vi "_old_Load_SetList_Convert_v4.0_to_v4.1.vi"(0 "Path":path) -> (1 "Procedure Name":string="IBS_PICameraTest_29Sep04", 2 "Paramaters":T1={"Master PB Staging List"=[{"Output Bits"=[], "Delay (s)"="", "String"="", "Halt?"=FALSE}, {"Output Bits"=[], "Delay (s)"="", "String"="", "Halt?"=FALSE}, {"Output Bits"=[], "Delay (s)"="", "String"="", "Halt?"=FALSE}, {"Output Bits"=[], "Delay (s)"="", "String"="", "Halt?"=FALSE}, {"Output Bits"=[], "Delay (s)"="", "String"="", "Halt?"=FALSE}, {"Output Bits"=[], "Delay (s)"="", "String"="", "Halt?"=FALSE}, {"Output Bits"=[], "Delay (s)"="", "String"="", "Halt?"=FALSE}, {"Output Bits"=[], "Delay (s)"="", "String"="", "Halt?"=FALSE}, {"Output Bits"=[], "Delay (s)"="", "String"="", "Halt?"=FALSE}, {"Output Bits"=[], "Delay (s)"="", "String"="", "Halt?"=FALSE}, {"Output Bits"=[], "Delay (s)"="", "String"="", "Halt?"=FALSE}, {"Output Bits"=[], "Delay (s)"="", "String"="", "Halt?"=FALSE}, {"Output Bits"=[], "Delay (s)"="", "String"="", "Halt?"=FALSE}, {"Output Bits"=[], "Delay (s)"="", "String"="", "Halt?"=FALSE}, {"Output Bits"=[], "Delay (s)"="", "String"="", "Halt?"=FALSE}, {"Output Bits"=[], "Delay (s)"="", "String"="", "Halt?"=FALSE}, {"Output Bits"=[], "Delay (s)"="", "String"="", "Halt?"=FALSE}, {"Output Bits"=[], "Delay (s)"="", "String"="", "Halt?"=FALSE}, {"Output Bits"=[], "Delay (s)"="", "String"="", "Halt?"=FALSE}, {"Output Bits"=[], "Delay (s)"="", "String"="", "Halt?"=FALSE}, {"Output Bits"=[], "Delay (s)"="", "String"="", "Halt?"=FALSE}, {"Output Bits"=[], "Delay (s)"="", "String"="", "Halt?"=FALSE}, {"Output Bits"=[], "Delay (s)"="", "String"="", "Halt?"=FALSE}, {"Output Bits"=[], "Delay (s)"="", "String"="", "Halt?"=FALSE}, {"Output Bits"=[], "Delay (s)"="", "String"="", "Halt?"=FALSE}, {"Output Bits"=[], "Delay (s)"="", "String"="", "Halt?"=FALSE}, {"Output Bits"=[], "Delay (s)"="", "String"="", "Halt?"=FALSE}, {"Output Bits"=[], "Delay (s)"="", "String"="", "Halt?"=FALSE}, {"Output Bits"=[], "Delay (s)"="", "String"="", "Halt?"=FALSE}, {"Output Bits"=[], "Delay (s)"="", "String"="", "Halt?"=FALSE}, {"Output Bits"=[], "Delay (s)"="", "String"="", "Halt?"=FALSE}, {"Output Bits"=[], "Delay (s)"="", "String"="", "Halt?"=FALSE}, {"Output Bits"=[], "Delay (s)"="", "String"="", "Halt?"=FALSE}, {"Output Bits"=[], "Delay (s)"="", "String"="", "Halt?"=FALSE}, {"Output Bits"=[], "Delay (s)"="", "String"="", "Halt?"=FALSE}, {"Output Bits"=[], "Delay (s)"="", "String"="", "Halt?"=FALSE}, {"Output Bits"=[], "Delay (s)"="", "String"="", "Halt?"=FALSE}, {"Output Bits"=[], "Delay (s)"="", "String"="", "Halt?"=FALSE}, {"Output Bits"=[], "Delay (s)"="", "String"="", "Halt?"=FALSE}, {"Output Bits"=[], "Delay (s)"="", "String"="", "Halt?"=FALSE}, {"Output Bits"=[], "Delay (s)"="", "String"="", "Halt?"=FALSE}, {"Output Bits"=[], "Delay (s)"="", "String"="", "Halt?"=FALSE}, {"Output Bits"=[], "Delay (s)"="", "String"="", "Halt?"=FALSE}, {"Output Bits"=[], "Delay (s)"="", "String"="", "Halt?"=FALSE}], "Slave PB Staging List"=[{"Output Bits"=[], "Delay (s)"="", "String"="", "Halt?"=FALSE}, {"Output Bits"=[], "Delay (s)"="", "String"="", "Halt?"=FALSE}, {"Output Bits"=[], "Delay (s)"="", "String"="", "Halt?"=FALSE}, {"Output Bits"=[], "Delay (s)"="", "String"="", "Halt?"=FALSE}, {"Output Bits"=[], "Delay (s)"="", "String"="", "Halt?"=FALSE}, {"Output Bits"=[], "Delay (s)"="", "String"="", "Halt?"=FALSE}, {"Output Bits"=[], "Delay (s)"="", "String"="", "Halt?"=FALSE}, {"Output Bits"=[], "Delay (s)"="", "String"="", "Halt?"=FALSE}, {"Output Bits"=[], "Delay (s)"="", "String"="", "Halt?"=FALSE}, {"Output Bits"=[], "Delay (s)"="", "String"="", "Halt?"=FALSE}, {"Output Bits"=[], "Delay (s)"="", "String"="", "Halt?"=FALSE}, {"Output Bits"=[], "Delay (s)"="", "String"="", "Halt?"=FALSE}, {"Output Bits"=[], "Delay (s)"="", "String"="", "Halt?"=FALSE}, {"Output Bits"=[], "Delay (s)"="", "String"="", "Halt?"=FALSE}, {"Output Bits"=[], "Delay (s)"="", "String"="", "Halt?"=FALSE}, {"Output Bits"=[], "Delay (s)"="", "String"="", "Halt?"=FALSE}, {"Output Bits"=[], "Delay (s)"="", "String"="", "Halt?"=FALSE}, {"Output Bits"=[], "Delay (s)"="", "String"="", "Halt?"=FALSE}, {"Output Bits"=[], "Delay (s)"="", "String"="", "Halt?"=FALSE}, {"Output Bits"=[], "Delay (s)"="", "String"="", "Halt?"=FALSE}, {"Output Bits"=[], "Delay (s)"="", "String"="", "Halt?"=FALSE}, {"Output Bits"=[], "Delay (s)"="", "String"="", "Halt?"=FALSE}, {"Output Bits"=[], "Delay (s)"="", "String"="", "Halt?"=FALSE}, {"Output Bits"=[], "Delay (s)"="", "String"="", "Halt?"=FALSE}, {"Output Bits"=[], "Delay (s)"="", "String"="", "Halt?"=FALSE}, {"Output Bits"=[], "Delay (s)"="", "String"="", "Halt?"=FALSE}, {"Output Bits"=[], "Delay (s)"="", "String"="", "Halt?"=FALSE}, {"Output Bits"=[], "Delay (s)"="", "String"="", "Halt?"=FALSE}, {"Output Bits"=[], "Delay (s)"="", "String"="", "Halt?"=FALSE}, {"Output Bits"=[], "Delay (s)"="", "String"="", "Halt?"=FALSE}, {"Output Bits"=[], "Delay (s)"="", "String"="", "Halt?"=FALSE}, {"Output Bits"=[], "Delay (s)"="", "String"="", "Halt?"=FALSE}, {"Output Bits"=[], "Delay (s)"="", "String"="", "Halt?"=FALSE}, {"Output Bits"=[], "Delay (s)"="", "String"="", "Halt?"=FALSE}, {"Output Bits"=[], "Delay (s)"="", "String"="", "Halt?"=FALSE}, {"Output Bits"=[], "Delay (s)"="", "String"="", "Halt?"=FALSE}, {"Output Bits"=[], "Delay (s)"="", "String"="", "Halt?"=FALSE}, {"Output Bits"=[], "Delay (s)"="", "String"="", "Halt?"=FALSE}, {"Output Bits"=[], "Delay (s)"="", "String"="", "Halt?"=FALSE}, {"Output Bits"=[], "Delay (s)"="", "String"="", "Halt?"=FALSE}, {"Output Bits"=[], "Delay (s)"="", "String"="", "Halt?"=FALSE}, {"Output Bits"=[], "Delay (s)"="", "String"="", "Halt?"=FALSE}, {"Output Bits"=[], "Delay (s)"="", "String"="", "Halt?"=FALSE}, {"Output Bits"=[], "Delay (s)"="", "String"="", "Halt?"=FALSE}], "Novatech Ramps"=[{"Ramp Channels"=[], "2 Freq. [MHz]"="", "2 Power [dBm]"="", "3 Freq. [MHz]"="", "3 Power [dBm]"="", "Serial Port"=""}, {"Ramp Channels"=[], "2 Freq. [MHz]"="", "2 Power [dBm]"="", "3 Freq. [MHz]"="", "3 Power [dBm]"="", "Serial Port"=""}, {"Ramp Channels"=[], "2 Freq. [MHz]"="", "2 Power [dBm]"="", "3 Freq. [MHz]"="", "3 Power [dBm]"="", "Serial Port"=""}, {"Ramp Channels"=[], "2 Freq. [MHz]"="", "2 Power [dBm]"="", "3 Freq. [MHz]"="", "3 Power [dBm]"="", "Serial Port"=""}, {"Ramp Channels"=[], "2 Freq. [MHz]"="", "2 Power [dBm]"="", "3 Freq. [MHz]"="", "3 Power [dBm]"="", "Serial Port"=""}, {"Ramp Channels"=[], "2 Freq. [MHz]"="", "2 Power [dBm]"="", "3 Freq. [MHz]"="", "3 Power [dBm]"="", "Serial Port"=""}, {"Ramp Channels"=[], "2 Freq. [MHz]"="", "2 Power [dBm]"="", "3 Freq. [MHz]"="", "3 Power [dBm]"="", "Serial Port"=""}], "Sequencing Info"=[{"Start"=0.0, "End"=2.11, "Sequenced Data"=[], "Inform\nIgor?"=FALSE, "Computed Step Size"=0.0, "Procedure Variable"="", "Default"=2.11, "Steps"=0}], "SRS Ramps"=[{"lattice ramp"=[{"dt"="", "formula"=""}, {"dt"="", "formula"=""}, {"dt"="", "formula"=""}], "Output"=[{"Time Values"=[0.0, 0.002, 0.004, 0.006, 0.008, 0.01, 0.012, 0.014, 0.016, 0.018000000000000002, 0.02, 0.022, 0.024, 0.026000000000000002, 0.028, 0.03, 0.032, 0.034, 0.036000000000000004, 0.038, 0.04, 0.042, 0.044, 0.046, 0.048, 0.05, 0.052000000000000005, 0.054, 0.056, 0.058, 0.06, 0.062, 0.064, 0.066, 0.068, 0.07, 0.07200000000000001, 0.074, 0.076, 0.078, 0.08, 0.082, 0.084, 0.08600000000000001, 0.088, 0.09, 0.092, 0.094, 0.096, 0.098, 0.1, 0.10200000000000001, 0.10400000000000001, 0.106, 0.108, 0.11, 0.112, 0.114, 0.116, 0.11800000000000001, 0.12, 0.122, 0.124, 0.126, 0.128, 0.13, 0.132, 0.134, 0.136, 0.138, 0.14, 0.14200000000000002, 0.14400000000000002, 0.146, 0.148, 0.15, 0.152, 0.154, 0.156, 0.158, 0.16, 0.162, 0.164, 0.166, 0.168, 0.17, 0.17200000000000001, 0.17400000000000002, 0.176, 0.178, 0.18, 0.182, 0.184, 0.186, 0.188, 0.19, 0.192, 0.194, 0.196, 0.198, 0.2, 0.6000000000000001, 0.6000000000000001, 0.6002000000000001, 0.6004, 0.6006000000000001, 0.6008000000000001, 0.6010000000000001, 0.6012000000000001, 0.6014, 0.6016000000000001, 0.6018000000000001, 0.6020000000000001, 0.6022000000000001, 0.6024, 0.6026000000000001, 0.6028000000000001, 0.6030000000000001, 0.6032000000000001, 0.6034, 0.6036000000000001, 0.6038000000000001, 0.6040000000000001, 0.6042000000000001, 0.6044, 0.6046000000000001, 0.6048000000000001, 0.6050000000000001, 0.6052000000000001, 0.6054, 0.6056000000000001, 0.6058000000000001, 0.6060000000000001, 0.6062000000000001, 0.6064, 0.6066000000000001, 0.6068000000000001, 0.6070000000000001, 0.6072000000000001, 0.6074, 0.6076000000000001, 0.6078000000000001, 0.6080000000000001, 0.6082000000000001, 0.6084, 0.6086000000000001, 0.6088000000000001, 0.6090000000000001, 0.6092000000000001, 0.6094, 0.6096000000000001, 0.6098000000000001, 0.6100000000000001, 0.6102000000000001, 0.6104, 0.6106000000000001, 0.6108000000000001, 0.6110000000000001, 0.6112000000000001, 0.6114, 0.6116000000000001, 0.6118000000000001, 0.6120000000000001, 0.6122000000000001, 0.6124, 0.6126, 0.6128000000000001, 0.6130000000000001, 0.6132000000000001, 0.6134000000000001, 0.6136000000000001, 0.6138000000000001, 0.6140000000000001, 0.6142000000000001, 0.6144000000000001, 0.6146, 0.6148000000000001, 0.6150000000000001, 0.6152000000000001, 0.6154000000000001, 0.6156, 0.6158000000000001, 0.6160000000000001, 0.6162000000000001, 0.6164000000000001, 0.6166, 0.6168000000000001, 0.6170000000000001, 0.6172000000000001, 0.6174000000000001, 0.6176, 0.6178000000000001, 0.6180000000000001, 0.6182000000000001, 0.6184000000000001, 0.6186, 0.6188000000000001, 0.6190000000000001, 0.6192000000000001, 0.6194000000000001, 0.6196, 0.6198000000000001, 0.6200000000000001, 0.6202000000000001, 0.6212000000000001], array[205 elements]}, {"Time Values"=[0.0, 0.002, 0.004, 0.006, 0.008, 0.01, 0.012, 0.014, 0.016, 0.018000000000000002, 0.02, 0.022, 0.024, 0.026000000000000002, 0.028, 0.03, 0.032, 0.034, 0.036000000000000004, 0.038, 0.04, 0.042, 0.044, 0.046, 0.048, 0.05, 0.052000000000000005, 0.054, 0.056, 0.058, 0.06, 0.062, 0.064, 0.066, 0.068, 0.07, 0.07200000000000001, 0.074, 0.076, 0.078, 0.08, 0.082, 0.084, 0.08600000000000001, 0.088, 0.09, 0.092, 0.094, 0.096, 0.098, 0.1, 0.10200000000000001, 0.10400000000000001, 0.106, 0.108, 0.11, 0.112, 0.114, 0.116, 0.11800000000000001, 0.12, 0.122, 0.124, 0.126, 0.128, 0.13, 0.132, 0.134, 0.136, 0.138, 0.14, 0.14200000000000002, 0.14400000000000002, 0.146, 0.148, 0.15, 0.152, 0.154, 0.156, 0.158, 0.16, 0.162, 0.164, 0.166, 0.168, 0.17, 0.17200000000000001, 0.17400000000000002, 0.176, 0.178, 0.18, 0.182, 0.184, 0.186, 0.188, 0.19, 0.192, 0.194, 0.196, 0.198, 0.2, 0.6000000000000001, 0.6000000000000001, 0.6002000000000001, 0.6004, 0.6006000000000001, 0.6008000000000001, 0.6010000000000001, 0.6012000000000001, 0.6014, 0.6016000000000001, 0.6018000000000001, 0.6020000000000001, 0.6022000000000001, 0.6024, 0.6026000000000001, 0.6028000000000001, 0.6030000000000001, 0.6032000000000001, 0.6034, 0.6036000000000001, 0.6038000000000001, 0.6040000000000001, 0.6042000000000001, 0.6044, 0.6046000000000001, 0.6048000000000001, 0.6050000000000001, 0.6052000000000001, 0.6054, 0.6056000000000001, 0.6058000000000001, 0.6060000000000001, 0.6062000000000001, 0.6064, 0.6066000000000001, 0.6068000000000001, 0.6070000000000001, 0.6072000000000001, 0.6074, 0.6076000000000001, 0.6078000000000001, 0.6080000000000001, 0.6082000000000001, 0.6084, 0.6086000000000001, 0.6088000000000001, 0.6090000000000001, 0.6092000000000001, 0.6094, 0.6096000000000001, 0.6098000000000001, 0.6100000000000001, 0.6102000000000001, 0.6104, 0.6106000000000001, 0.6108000000000001, 0.6110000000000001, 0.6112000000000001, 0.6114, 0.6116000000000001, 0.6118000000000001, 0.6120000000000001, 0.6122000000000001, 0.6124, 0.6126, 0.6128000000000001, 0.6130000000000001, 0.6132000000000001, 0.6134000000000001, 0.6136000000000001, 0.6138000000000001, 0.6140000000000001, 0.6142000000000001, 0.6144000000000001, 0.6146, 0.6148000000000001, 0.6150000000000001, 0.6152000000000001, 0.6154000000000001, 0.6156, 0.6158000000000001, 0.6160000000000001, 0.6162000000000001, 0.6164000000000001, 0.6166, 0.6168000000000001, 0.6170000000000001, 0.6172000000000001, 0.6174000000000001, 0.6176, 0.6178000000000001, 0.6180000000000001, 0.6182000000000001, 0.6184000000000001, 0.6186, 0.6188000000000001, 0.6190000000000001, 0.6192000000000001, 0.6194000000000001, 0.6196, 0.6198000000000001, 0.6200000000000001, 0.6202000000000001, 0.6212000000000001], array[205 elements]}], "SRS Selection"=enum."1550 Vertical"}, {"lattice ramp"=[{"dt"="", "formula"=""}], "Output"=[{"Time Values"=[0.0, 0.002, 0.004, 0.006, 0.008, 0.01, 0.012, 0.014, 0.016, 0.018000000000000002, 0.02, 0.022, 0.024, 0.026000000000000002, 0.028, 0.03, 0.032, 0.034, 0.036000000000000004, 0.038, 0.04, 0.042, 0.044, 0.046, 0.048, 0.05, 0.052000000000000005, 0.054, 0.056, 0.058, 0.06, 0.062, 0.064, 0.066, 0.068, 0.07, 0.07200000000000001, 0.074, 0.076, 0.078, 0.08, 0.082, 0.084, 0.08600000000000001, 0.088, 0.09, 0.092, 0.094, 0.096, 0.098, 0.1, 0.10200000000000001, 0.10400000000000001, 0.106, 0.108, 0.11, 0.112, 0.114, 0.116, 0.11800000000000001, 0.12, 0.122, 0.124, 0.126, 0.128, 0.13, 0.132, 0.134, 0.136, 0.138, 0.14, 0.14200000000000002, 0.14400000000000002, 0.146, 0.148, 0.15, 0.152, 0.154, 0.156, 0.158, 0.16, 0.162, 0.164, 0.166, 0.168, 0.17, 0.17200000000000001, 0.17400000000000002, 0.176, 0.178, 0.18, 0.182, 0.184, 0.186, 0.188, 0.19, 0.192, 0.194, 0.196, 0.198, 0.2, 0.6000000000000001, 0.6000000000000001, 0.6002000000000001, 0.6004, 0.6006000000000001, 0.6008000000000001, 0.6010000000000001, 0.6012000000000001, 0.6014, 0.6016000000000001, 0.6018000000000001, 0.6020000000000001, 0.6022000000000001, 0.6024, 0.6026000000000001, 0.6028000000000001, 0.6030000000000001, 0.6032000000000001, 0.6034, 0.6036000000000001, 0.6038000000000001, 0.6040000000000001, 0.6042000000000001, 0.6044, 0.6046000000000001, 0.6048000000000001, 0.6050000000000001, 0.6052000000000001, 0.6054, 0.6056000000000001, 0.6058000000000001, 0.6060000000000001, 0.6062000000000001, 0.6064, 0.6066000000000001, 0.6068000000000001, 0.6070000000000001, 0.6072000000000001, 0.6074, 0.6076000000000001, 0.6078000000000001, 0.6080000000000001, 0.6082000000000001, 0.6084, 0.6086000000000001, 0.6088000000000001, 0.6090000000000001, 0.6092000000000001, 0.6094, 0.6096000000000001, 0.6098000000000001, 0.6100000000000001, 0.6102000000000001, 0.6104, 0.6106000000000001, 0.6108000000000001, 0.6110000000000001, 0.6112000000000001, 0.6114, 0.6116000000000001, 0.6118000000000001, 0.6120000000000001, 0.6122000000000001, 0.6124, 0.6126, 0.6128000000000001, 0.6130000000000001, 0.6132000000000001, 0.6134000000000001, 0.6136000000000001, 0.6138000000000001, 0.6140000000000001, 0.6142000000000001, 0.6144000000000001, 0.6146, 0.6148000000000001, 0.6150000000000001, 0.6152000000000001, 0.6154000000000001, 0.6156, 0.6158000000000001, 0.6160000000000001, 0.6162000000000001, 0.6164000000000001, 0.6166, 0.6168000000000001, 0.6170000000000001, 0.6172000000000001, 0.6174000000000001, 0.6176, 0.6178000000000001, 0.6180000000000001, 0.6182000000000001, 0.6184000000000001, 0.6186, 0.6188000000000001, 0.6190000000000001, 0.6192000000000001, 0.6194000000000001, 0.6196, 0.6198000000000001, 0.6200000000000001, 0.6202000000000001, 0.6212000000000001], array[205 elements]}, {"Time Values"=[0.0, 0.002, 0.004, 0.006, 0.008, 0.01, 0.012, 0.014, 0.016, 0.018000000000000002, 0.02, 0.022, 0.024, 0.026000000000000002, 0.028, 0.03, 0.032, 0.034, 0.036000000000000004, 0.038, 0.04, 0.042, 0.044, 0.046, 0.048, 0.05, 0.052000000000000005, 0.054, 0.056, 0.058, 0.06, 0.062, 0.064, 0.066, 0.068, 0.07, 0.07200000000000001, 0.074, 0.076, 0.078, 0.08, 0.082, 0.084, 0.08600000000000001, 0.088, 0.09, 0.092, 0.094, 0.096, 0.098, 0.1, 0.10200000000000001, 0.10400000000000001, 0.106, 0.108, 0.11, 0.112, 0.114, 0.116, 0.11800000000000001, 0.12, 0.122, 0.124, 0.126, 0.128, 0.13, 0.132, 0.134, 0.136, 0.138, 0.14, 0.14200000000000002, 0.14400000000000002, 0.146, 0.148, 0.15, 0.152, 0.154, 0.156, 0.158, 0.16, 0.162, 0.164, 0.166, 0.168, 0.17, 0.17200000000000001, 0.17400000000000002, 0.176, 0.178, 0.18, 0.182, 0.184, 0.186, 0.188, 0.19, 0.192, 0.194, 0.196, 0.198, 0.2, 0.6000000000000001, 0.6000000000000001, 0.6002000000000001, 0.6004, 0.6006000000000001, 0.6008000000000001, 0.6010000000000001, 0.6012000000000001, 0.6014, 0.6016000000000001, 0.6018000000000001, 0.6020000000000001, 0.6022000000000001, 0.6024, 0.6026000000000001, 0.6028000000000001, 0.6030000000000001, 0.6032000000000001, 0.6034, 0.6036000000000001, 0.6038000000000001, 0.6040000000000001, 0.6042000000000001, 0.6044, 0.6046000000000001, 0.6048000000000001, 0.6050000000000001, 0.6052000000000001, 0.6054, 0.6056000000000001, 0.6058000000000001, 0.6060000000000001, 0.6062000000000001, 0.6064, 0.6066000000000001, 0.6068000000000001, 0.6070000000000001, 0.6072000000000001, 0.6074, 0.6076000000000001, 0.6078000000000001, 0.6080000000000001, 0.6082000000000001, 0.6084, 0.6086000000000001, 0.6088000000000001, 0.6090000000000001, 0.6092000000000001, 0.6094, 0.6096000000000001, 0.6098000000000001, 0.6100000000000001, 0.6102000000000001, 0.6104, 0.6106000000000001, 0.6108000000000001, 0.6110000000000001, 0.6112000000000001, 0.6114, 0.6116000000000001, 0.6118000000000001, 0.6120000000000001, 0.6122000000000001, 0.6124, 0.6126, 0.6128000000000001, 0.6130000000000001, 0.6132000000000001, 0.6134000000000001, 0.6136000000000001, 0.6138000000000001, 0.6140000000000001, 0.6142000000000001, 0.6144000000000001, 0.6146, 0.6148000000000001, 0.6150000000000001, 0.6152000000000001, 0.6154000000000001, 0.6156, 0.6158000000000001, 0.6160000000000001, 0.6162000000000001, 0.6164000000000001, 0.6166, 0.6168000000000001, 0.6170000000000001, 0.6172000000000001, 0.6174000000000001, 0.6176, 0.6178000000000001, 0.6180000000000001, 0.6182000000000001, 0.6184000000000001, 0.6186, 0.6188000000000001, 0.6190000000000001, 0.6192000000000001, 0.6194000000000001, 0.6196, 0.6198000000000001, 0.6200000000000001, 0.6202000000000001, 0.6212000000000001], array[205 elements]}], "SRS Selection"=enum."1550 Vertical"}], "Master AO Ramp List"=[{"Ramp index"=10, "Ramp time [s]"="", "Step size [s]"=1000.0, "Ramp Array"=[], "Output Bits"=[]}, {"Ramp index"=10, "Ramp time [s]"="", "Step size [s]"=1000.0, "Ramp Array"=[], "Output Bits"=[]}], "Slave AO Ramp List"=[{"Ramp index"=10, "Ramp time [s]"="", "Step size [s]"=1000.0, "Ramp Array"=[], "Output Bits"=[]}, {"Ramp index"=10, "Ramp time [s]"="", "Step size [s]"=1000.0, "Ramp Array"=[], "Output Bits"=[]}], "Master Novatech Ramp List"=[], "Static Variables"=[], "DDS Ramp List"=[]} {"Sequencing Info"."Steps" min=2; "Sequencing Info"."Default" format="%#.7p"; "Sequencing Info"."Computed Step Size" format="%#.7p"; "Sequencing Info"."Sequenced Data" format="%.2e"; "Sequencing Info"."End" format="%#.7p"; "Sequencing Info"."Start" format="%#.7p"})   [LabVIEW 2013]
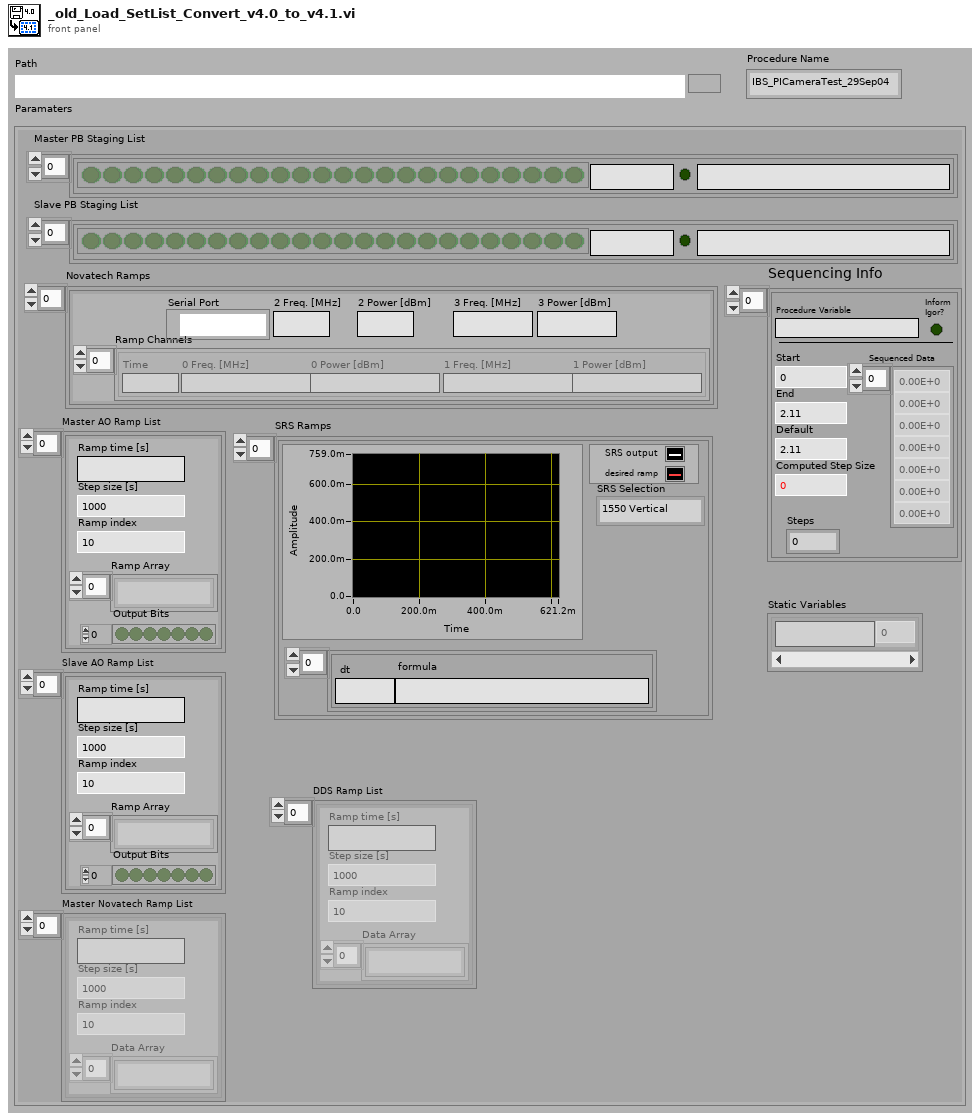
[diagram p1: front panel]
types:
  T1 = cluster{"Master PB Staging List":cluster{"Output Bits":bool[], "Delay (s)":string, "String":string, "Halt?":bool}[], "Slave PB Staging List":cluster{"Output Bits":bool[], "Delay (s)":string, "String":string, "Halt?":bool}[], "Novatech Ramps":cluster{"Ramp Channels":cluster{"Time":string, "0 Freq. [MHz]":string, "0 Power [dBm]":string, "1 Freq. [MHz]":string, "1 Power [dBm]":string}[], "2 Freq. [MHz]":string, "2 Power [dBm]":string, "3 Freq. [MHz]":string, "3 Power [dBm]":string, "Serial Port":refnum<visa-resource-name>}[], "Sequencing Info":cluster{"Start":dbl, "End":dbl, "Sequenced Data":dbl[], "Inform\nIgor?":bool, "Computed Step Size":dbl, "Procedure Variable":string, "Default":dbl, "Steps":i32}[], "SRS Ramps":cluster{"lattice ramp":cluster{"dt":string, "formula":string}[], "Output":cluster{"Time Values":dbl[], dbl[]}[], "SRS Selection":enum16{"1550 Vertical", "Bragg Agilent", "Bragg PTS", "Acc. Intensity"}}[], "Master AO Ramp List":cluster{"Ramp index":u32, "Ramp time [s]":string, "Step size [s]":dbl, "Ramp Array":string[], "Output Bits":bool[]}[], "Slave AO Ramp List":cluster{"Ramp index":u32, "Ramp time [s]":string, "Step size [s]":dbl, "Ramp Array":string[], "Output Bits":bool[]}[], "Master Novatech Ramp List":cluster{"Ramp index":u32, "Ramp time [s]":string, "Step size [s]":dbl, "Data Array":string[]}[], "Static Variables":cluster{"Procedure variable":string, "Value":dbl}[], "DDS Ramp List":cluster{"Ramp index":u32, "Ramp time [s]":string, "Step size [s]":dbl, "Data Array":string[]}[]}
  T2 = cluster{"Master PB Staging List":cluster{"Output Bits":bool[], "Delay (s)":string, "String":string, "Halt?":bool}[], "Slave PB Staging List":cluster{"Output Bits":bool[], "Delay (s)":string, "String":string, "Halt?":bool}[], "Novatech Ramps":cluster{"Ramp Channels":cluster{"Time":string, "0 Freq. [MHz]":string, "0 Power [dBm]":string, "1 Freq. [MHz]":string, "1 Power [dBm]":string}[], "2 Freq. [MHz]":string, "2 Power [dBm]":string, "3 Freq. [MHz]":string, "3 Power [dBm]":string, "Serial Port":refnum<visa-resource-name>}[], "Sequencing Info":cluster{"Start":dbl, "End":dbl, "Sequenced Data":dbl[], "Sequence Data Source":bool, "Inform\nIgor?":bool, "Computed Step Size":dbl, "Procedure Variable":string, "Default":dbl}[], "SRS Ramps":cluster{"lattice ramp":cluster{"dt":string, "formula":string}[], "Output":cluster{"Time Values":dbl[], dbl[]}[], "SRS Selection":enum16{"1550 Vertical", "Bragg Agilent", "Bragg PTS", "Acc. Intensity"}}[], "Master AO Ramp List":cluster{"Ramp index":u32, "Ramp time [s]":string, "Step size [s]":dbl, "Ramp Array":string[], "Output Bits":bool[]}[], "Slave AO Ramp List":cluster{"Ramp index":u32, "Ramp time [s]":string, "Step size [s]":dbl, "Ramp Array":string[], "Output Bits":bool[]}[], "Master Novatech Ramp List":cluster{"Ramp index":u32, "Ramp time [s]":string, "Step size [s]":dbl, "Data Array":string[]}[], "Static Variables":cluster{"Procedure variable":string, "Value":dbl}[]}
  T3 = cluster{"Output Bits":bool[], "Delay (s)":string, "String":string, "Halt?":bool}[]
  T4 = cluster{"Ramp index":u32, "Ramp time [s]":string, "Step size [s]":dbl, "Ramp Array":string[], "Output Bits":bool[]}[]
  T5 = cluster{"Ramp index":u32, "Ramp time [s]":string, "Step size [s]":dbl, "Data Array":string[]}[]
  T6 = cluster{"Ramp Channels":cluster{"Time":string, "0 Freq. [MHz]":string, "0 Power [dBm]":string, "1 Freq. [MHz]":string, "1 Power [dBm]":string}[], "2 Freq. [MHz]":string, "2 Power [dBm]":string, "3 Freq. [MHz]":string, "3 Power [dBm]":string, "Serial Port":refnum<visa-resource-name>}[]
  T7 = cluster{"Start":dbl, "End":dbl, "Sequenced Data":dbl[], "Sequence Data Source":bool, "Inform\nIgor?":bool, "Computed Step Size":dbl, "Procedure Variable":string, "Default":dbl}[]
  T8 = cluster{"lattice ramp":cluster{"dt":string, "formula":string}[], "Output":cluster{"Time Values":dbl[], dbl[]}[], "SRS Selection":enum16{"1550 Vertical", "Bragg Agilent", "Bragg PTS", "Acc. Intensity"}}[]
  T9 = cluster{"Procedure variable":string, "Value":dbl}[]
  T10 = cluster{"Ramp index":u32, "Ramp time [s]":string, "Step size [s]":dbl, "Ramp Array":string[], "Output Bits":bool[]}
  T11 = cluster{"Ramp index":u32, "Ramp time [s]":string, "Step size [s]":dbl, "Data Array":string[]}
  T12 = cluster{"Output Bits":bool[], "Delay (s)":string, "String":string, "Halt?":bool}
  T13 = cluster{"Ramp Channels":cluster{"Time":string, "0 Freq. [MHz]":string, "0 Power [dBm]":string, "1 Freq. [MHz]":string, "1 Power [dBm]":string}[], "2 Freq. [MHz]":string, "2 Power [dBm]":string, "3 Freq. [MHz]":string, "3 Power [dBm]":string, "Serial Port":refnum<visa-resource-name>}
  T14 = cluster{"Start":dbl, "End":dbl, "Sequenced Data":dbl[], "Sequence Data Source":bool, "Inform\nIgor?":bool, "Computed Step Size":dbl, "Procedure Variable":string, "Default":dbl}
  T15 = cluster{"Start":dbl, "End":dbl, "Sequenced Data":dbl[], "Inform\nIgor?":bool, "Computed Step Size":dbl, "Procedure Variable":string, "Default":dbl, "Steps":i32}
  T16 = cluster{"Procedure variable":string, "Value":dbl}
  T17 = cluster{"lattice ramp":cluster{"dt":string, "formula":string}[], "Output":cluster{"Time Values":dbl[], dbl[]}[], "SRS Selection":enum16{"1550 Vertical", "Bragg Agilent", "Bragg PTS", "Acc. Intensity"}}
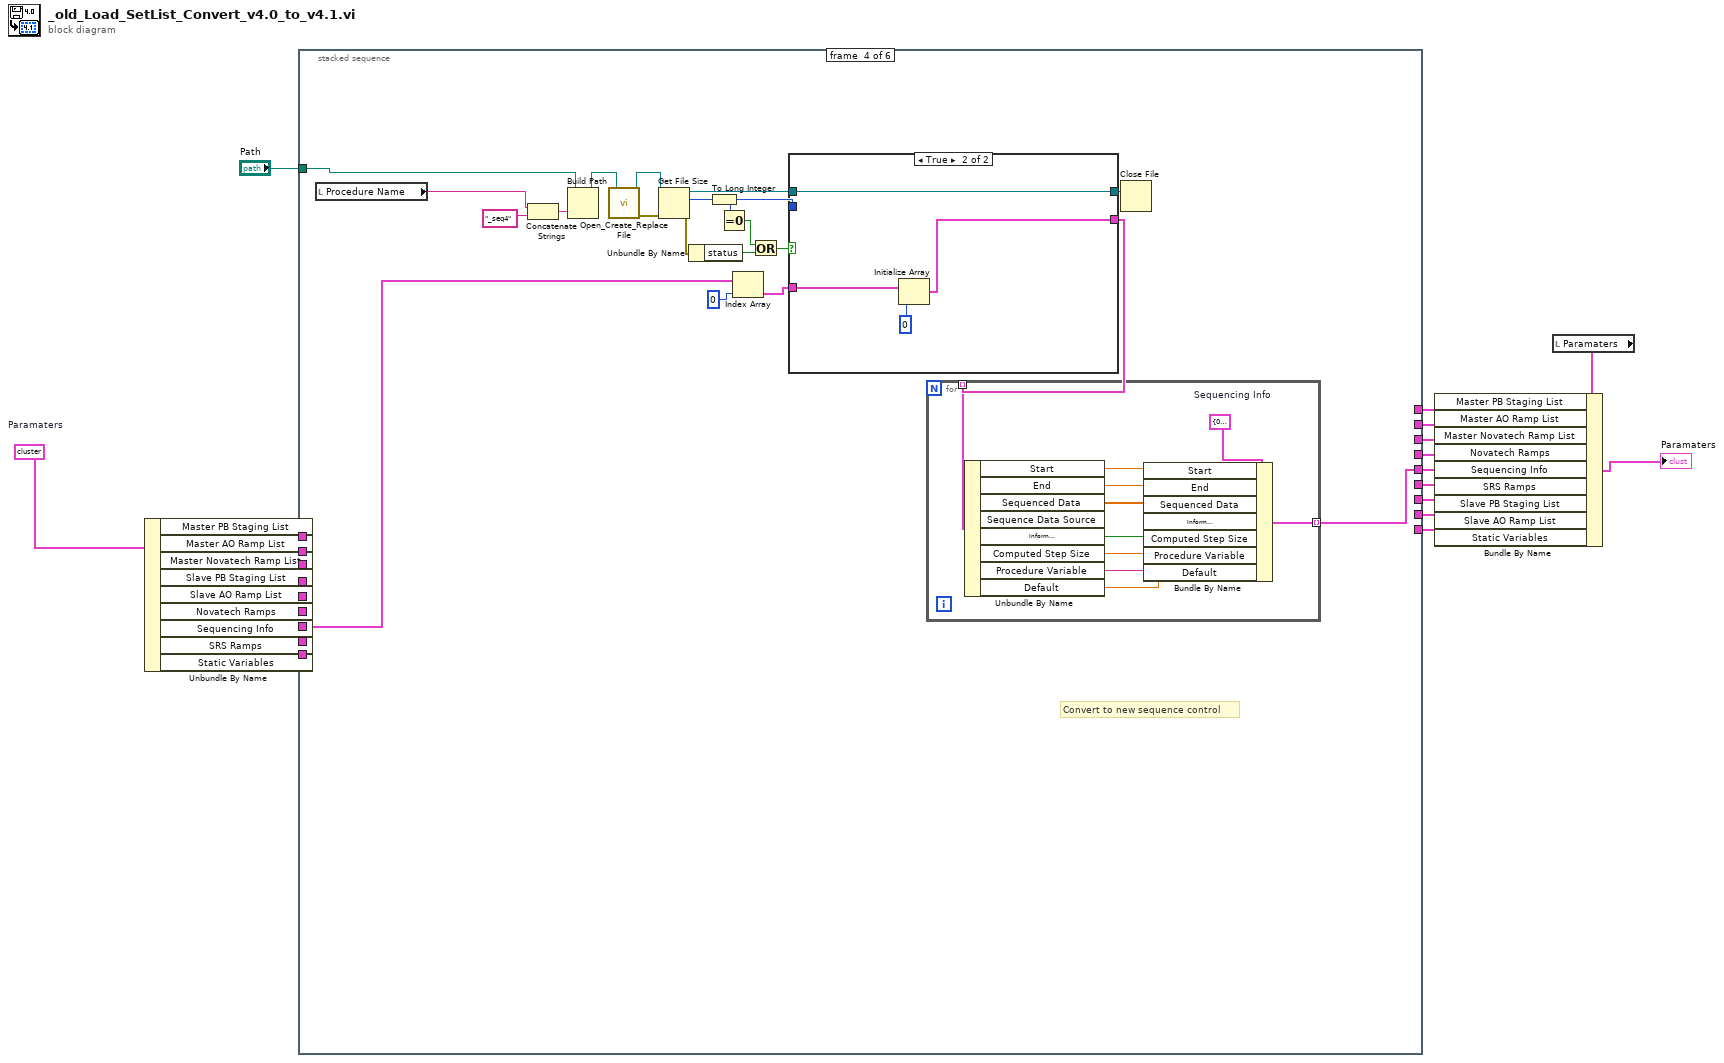
[diagram p0: block diagram]
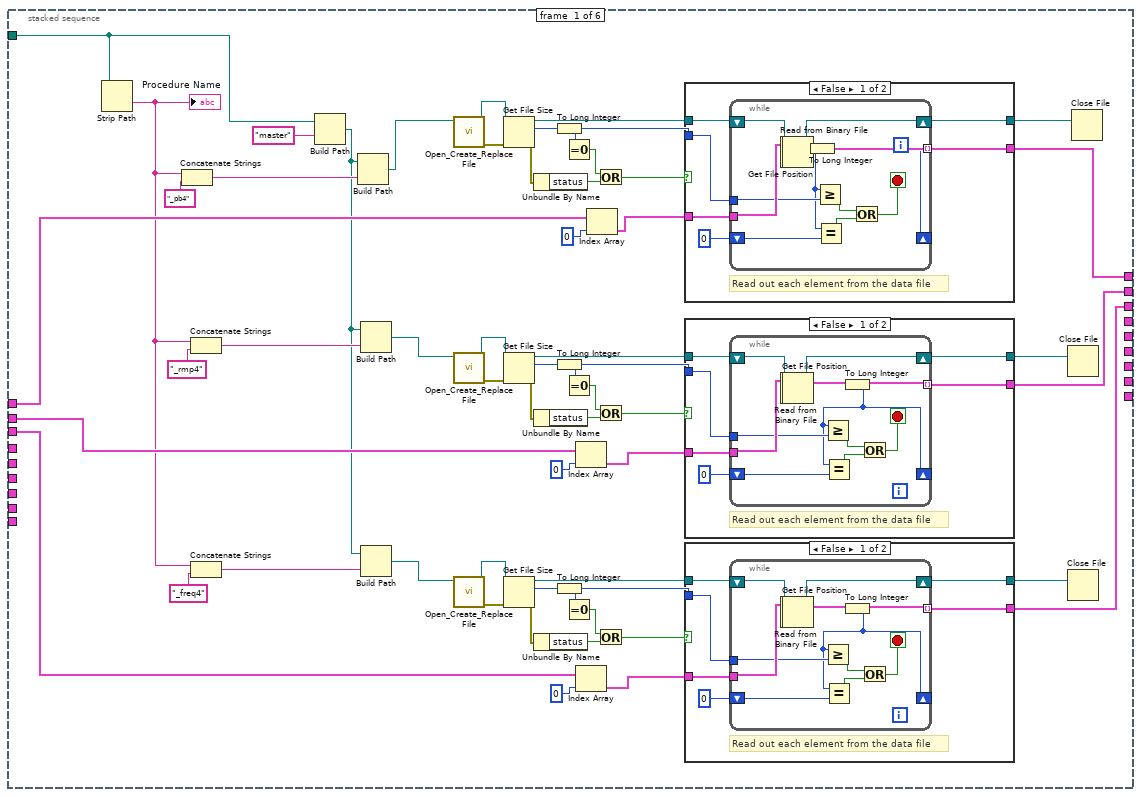
[diagram p2: hidden frame]
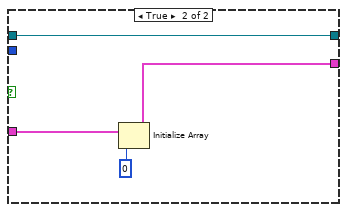
[diagram p3: hidden frame]
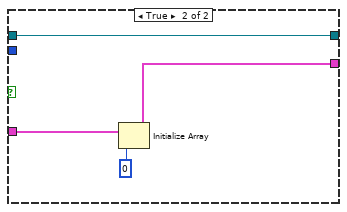
[diagram p4: hidden frame]
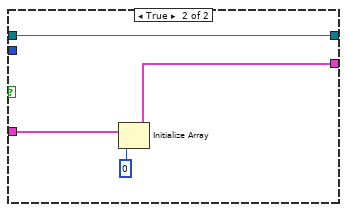
[diagram p5: hidden frame]
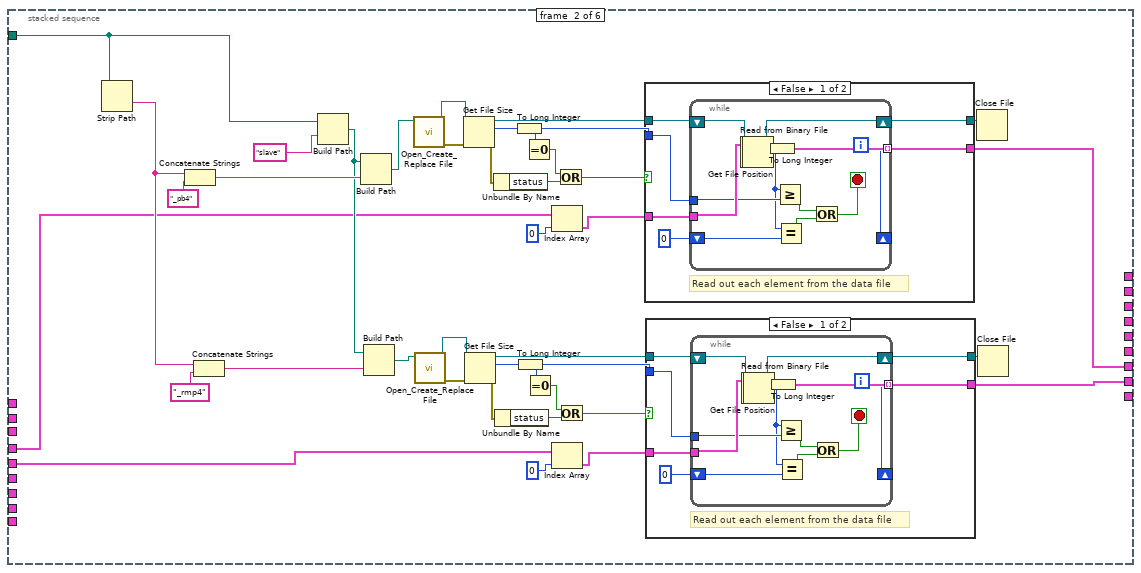
[diagram p6: hidden frame]
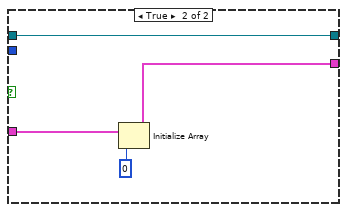
[diagram p7: hidden frame]
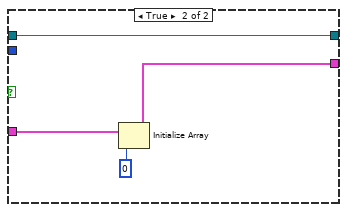
[diagram p8: hidden frame]
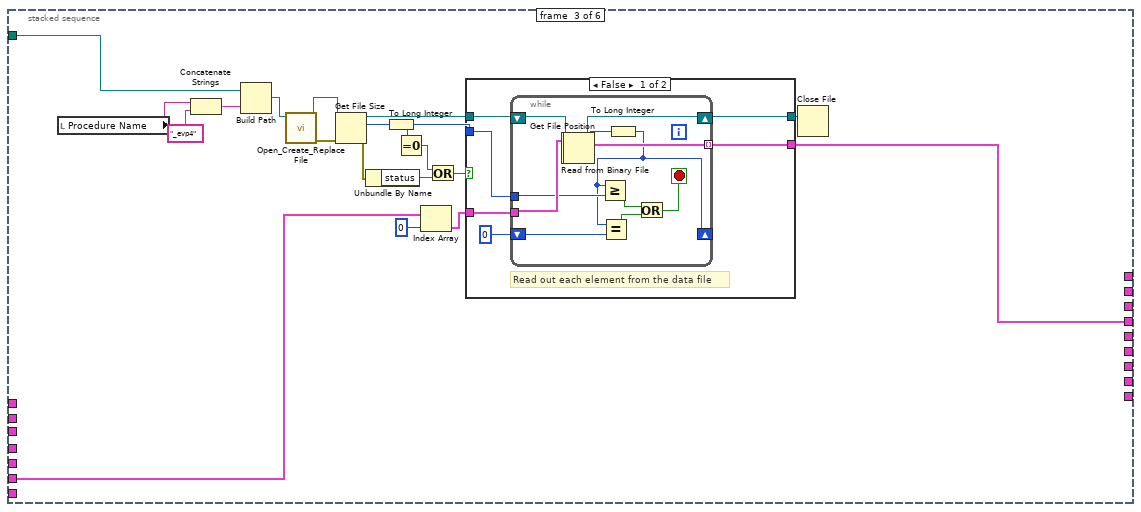
[diagram p9: hidden frame]
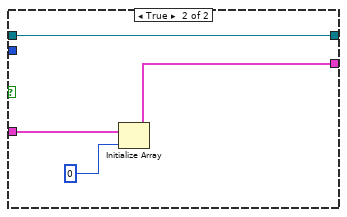
[diagram p10: hidden frame]
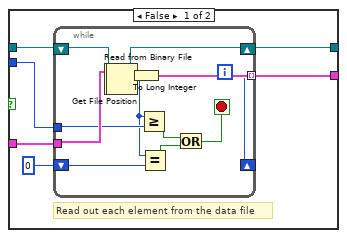
[diagram p11: hidden frame]
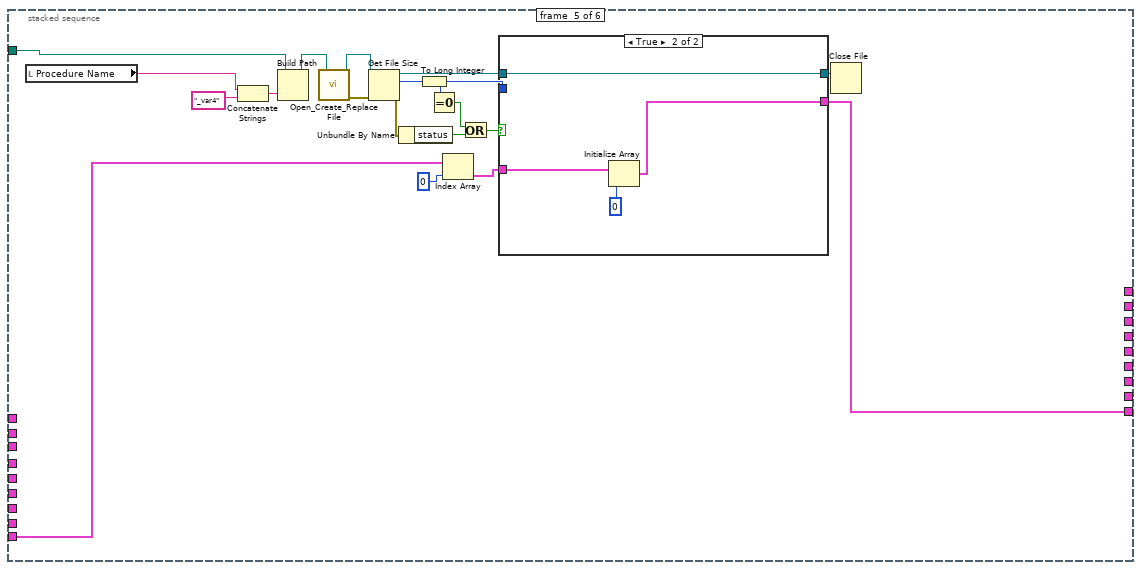
[diagram p12: hidden frame]
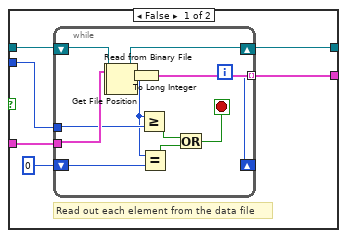
[diagram p13: hidden frame]
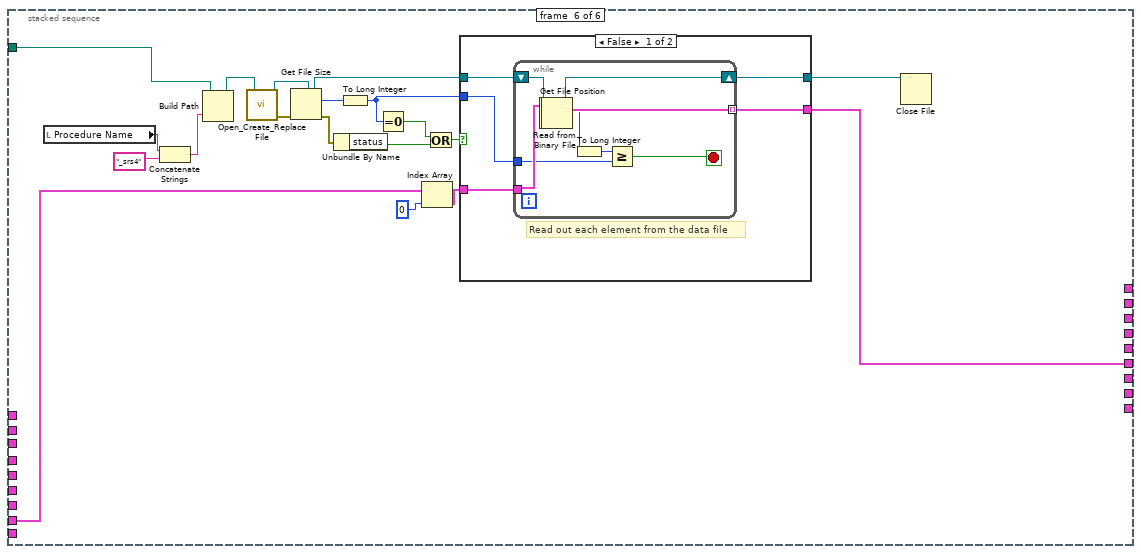
[diagram p14: hidden frame]
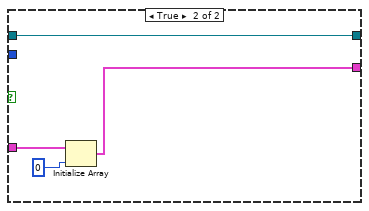
[diagram p15: hidden frame]
diagram:
  w1 = T2 {"Master PB Staging List"=[{"Output Bits"=[], "Delay (s)"="", "String"="", "Halt?"=FALSE}, {"Output Bits"=[], "Delay (s)"="", "String"="", "Halt?"=FALSE}, {"Output Bits"=[], "Delay (s)"="", "String"="", "Halt?"=FALSE}, {"Output Bits"=[], "Delay (s)"="", "String"="", "Halt?"=FALSE}, {"Output Bits"=[], "Delay (s)"="", "String"="", "Halt?"=FALSE}, {"Output Bits"=[], "Delay (s)"="", "String"="", "Halt?"=FALSE}, {"Output Bits"=[], "Delay (s)"="", "String"="", "Halt?"=FALSE}, {"Output Bits"=[], "Delay (s)"="", "String"="", "Halt?"=FALSE}, {"Output Bits"=[], "Delay (s)"="", "String"="", "Halt?"=FALSE}, {"Output Bits"=[], "Delay (s)"="", "String"="", "Halt?"=FALSE}, {"Output Bits"=[], "Delay (s)"="", "String"="", "Halt?"=FALSE}, {"Output Bits"=[], "Delay (s)"="", "String"="", "Halt?"=FALSE}, {"Output Bits"=[], "Delay (s)"="", "String"="", "Halt?"=FALSE}, {"Output Bits"=[], "Delay (s)"="", "String"="", "Halt?"=FALSE}, {"Output Bits"=[], "Delay (s)"="", "String"="", "Halt?"=FALSE}, {"Output Bits"=[], "Delay (s)"="", "String"="", "Halt?"=FALSE}, {"Output Bits"=[], "Delay (s)"="", "String"="", "Halt?"=FALSE}, {"Output Bits"=[], "Delay (s)"="", "String"="", "Halt?"=FALSE}, {"Output Bits"=[], "Delay (s)"="", "String"="", "Halt?"=FALSE}, {"Output Bits"=[], "Delay (s)"="", "String"="", "Halt?"=FALSE}, {"Output Bits"=[], "Delay (s)"="", "String"="", "Halt?"=FALSE}, {"Output Bits"=[], "Delay (s)"="", "String"="", "Halt?"=FALSE}, {"Output Bits"=[], "Delay (s)"="", "String"="", "Halt?"=FALSE}, {"Output Bits"=[], "Delay (s)"="", "String"="", "Halt?"=FALSE}, {"Output Bits"=[], "Delay (s)"="", "String"="", "Halt?"=FALSE}, {"Output Bits"=[], "Delay (s)"="", "String"="", "Halt?"=FALSE}, {"Output Bits"=[], "Delay (s)"="", "String"="", "Halt?"=FALSE}, {"Output Bits"=[], "Delay (s)"="", "String"="", "Halt?"=FALSE}, {"Output Bits"=[], "Delay (s)"="", "String"="", "Halt?"=FALSE}, {"Output Bits"=[], "Delay (s)"="", "String"="", "Halt?"=FALSE}, {"Output Bits"=[], "Delay (s)"="", "String"="", "Halt?"=FALSE}, {"Output Bits"=[], "Delay (s)"="", "String"="", "Halt?"=FALSE}, {"Output Bits"=[], "Delay (s)"="", "String"="", "Halt?"=FALSE}, {"Output Bits"=[], "Delay (s)"="", "String"="", "Halt?"=FALSE}, {"Output Bits"=[], "Delay (s)"="", "String"="", "Halt?"=FALSE}, {"Output Bits"=[], "Delay (s)"="", "String"="", "Halt?"=FALSE}, {"Output Bits"=[], "Delay (s)"="", "String"="", "Halt?"=FALSE}, {"Output Bits"=[], "Delay (s)"="", "String"="", "Halt?"=FALSE}, {"Output Bits"=[], "Delay (s)"="", "String"="", "Halt?"=FALSE}, {"Output Bits"=[], "Delay (s)"="", "String"="", "Halt?"=FALSE}, {"Output Bits"=[], "Delay (s)"="", "String"="", "Halt?"=FALSE}, {"Output Bits"=[], "Delay (s)"="", "String"="", "Halt?"=FALSE}, {"Output Bits"=[], "Delay (s)"="", "String"="", "Halt?"=FALSE}, {"Output Bits"=[], "Delay (s)"="", "String"="", "Halt?"=FALSE}], "Slave PB Staging List"=[{"Output Bits"=[], "Delay (s)"="", "String"="", "Halt?"=FALSE}, {"Output Bits"=[], "Delay (s)"="", "String"="", "Halt?"=FALSE}, {"Output Bits"=[], "Delay (s)"="", "String"="", "Halt?"=FALSE}, {"Output Bits"=[], "Delay (s)"="", "String"="", "Halt?"=FALSE}, {"Output Bits"=[], "Delay (s)"="", "String"="", "Halt?"=FALSE}, {"Output Bits"=[], "Delay (s)"="", "String"="", "Halt?"=FALSE}, {"Output Bits"=[], "Delay (s)"="", "String"="", "Halt?"=FALSE}, {"Output Bits"=[], "Delay (s)"="", "String"="", "Halt?"=FALSE}, {"Output Bits"=[], "Delay (s)"="", "String"="", "Halt?"=FALSE}, {"Output Bits"=[], "Delay (s)"="", "String"="", "Halt?"=FALSE}, {"Output Bits"=[], "Delay (s)"="", "String"="", "Halt?"=FALSE}, {"Output Bits"=[], "Delay (s)"="", "String"="", "Halt?"=FALSE}, {"Output Bits"=[], "Delay (s)"="", "String"="", "Halt?"=FALSE}, {"Output Bits"=[], "Delay (s)"="", "String"="", "Halt?"=FALSE}, {"Output Bits"=[], "Delay (s)"="", "String"="", "Halt?"=FALSE}, {"Output Bits"=[], "Delay (s)"="", "String"="", "Halt?"=FALSE}, {"Output Bits"=[], "Delay (s)"="", "String"="", "Halt?"=FALSE}, {"Output Bits"=[], "Delay (s)"="", "String"="", "Halt?"=FALSE}, {"Output Bits"=[], "Delay (s)"="", "String"="", "Halt?"=FALSE}, {"Output Bits"=[], "Delay (s)"="", "String"="", "Halt?"=FALSE}, {"Output Bits"=[], "Delay (s)"="", "String"="", "Halt?"=FALSE}, {"Output Bits"=[], "Delay (s)"="", "String"="", "Halt?"=FALSE}, {"Output Bits"=[], "Delay (s)"="", "String"="", "Halt?"=FALSE}, {"Output Bits"=[], "Delay (s)"="", "String"="", "Halt?"=FALSE}, {"Output Bits"=[], "Delay (s)"="", "String"="", "Halt?"=FALSE}, {"Output Bits"=[], "Delay (s)"="", "String"="", "Halt?"=FALSE}, {"Output Bits"=[], "Delay (s)"="", "String"="", "Halt?"=FALSE}, {"Output Bits"=[], "Delay (s)"="", "String"="", "Halt?"=FALSE}, {"Output Bits"=[], "Delay (s)"="", "String"="", "Halt?"=FALSE}, {"Output Bits"=[], "Delay (s)"="", "String"="", "Halt?"=FALSE}, {"Output Bits"=[], "Delay (s)"="", "String"="", "Halt?"=FALSE}, {"Output Bits"=[], "Delay (s)"="", "String"="", "Halt?"=FALSE}, {"Output Bits"=[], "Delay (s)"="", "String"="", "Halt?"=FALSE}, {"Output Bits"=[], "Delay (s)"="", "String"="", "Halt?"=FALSE}, {"Output Bits"=[], "Delay (s)"="", "String"="", "Halt?"=FALSE}, {"Output Bits"=[], "Delay (s)"="", "String"="", "Halt?"=FALSE}, {"Output Bits"=[], "Delay (s)"="", "String"="", "Halt?"=FALSE}, {"Output Bits"=[], "Delay (s)"="", "String"="", "Halt?"=FALSE}, {"Output Bits"=[], "Delay (s)"="", "String"="", "Halt?"=FALSE}, {"Output Bits"=[], "Delay (s)"="", "String"="", "Halt?"=FALSE}, {"Output Bits"=[], "Delay (s)"="", "String"="", "Halt?"=FALSE}, {"Output Bits"=[], "Delay (s)"="", "String"="", "Halt?"=FALSE}, {"Output Bits"=[], "Delay (s)"="", "String"="", "Halt?"=FALSE}, {"Output Bits"=[], "Delay (s)"="", "String"="", "Halt?"=FALSE}], "Novatech Ramps"=[{"Ramp Channels"=[], "2 Freq. [MHz]"="", "2 Power [dBm]"="", "3 Freq. [MHz]"="", "3 Power [dBm]"="", "Serial Port"=""}, {"Ramp Channels"=[], "2 Freq. [MHz]"="", "2 Power [dBm]"="", "3 Freq. [MHz]"="", "3 Power [dBm]"="", "Serial Port"=""}, {"Ramp Channels"=[], "2 Freq. [MHz]"="", "2 Power [dBm]"="", "3 Freq. [MHz]"="", "3 Power [dBm]"="", "Serial Port"=""}, {"Ramp Channels"=[], "2 Freq. [MHz]"="", "2 Power [dBm]"="", "3 Freq. [MHz]"="", "3 Power [dBm]"="", "Serial Port"=""}, {"Ramp Channels"=[], "2 Freq. [MHz]"="", "2 Power [dBm]"="", "3 Freq. [MHz]"="", "3 Power [dBm]"="", "Serial Port"=""}, {"Ramp Channels"=[], "2 Freq. [MHz]"="", "2 Power [dBm]"="", "3 Freq. [MHz]"="", "3 Power [dBm]"="", "Serial Port"=""}, {"Ramp Channels"=[], "2 Freq. [MHz]"="", "2 Power [dBm]"="", "3 Freq. [MHz]"="", "3 Power [dBm]"="", "Serial Port"=""}], "Sequencing Info"=[{"Start"=0.0, "End"=2.11, "Sequenced Data"=[], "Sequence Data Source"=FALSE, "Inform\nIgor?"=FALSE, "Computed Step Size"=0.0, "Procedure Variable"="", "Default"=2.11}], "SRS Ramps"=[{"lattice ramp"=[{"dt"="", "formula"=""}, {"dt"="", "formula"=""}, {"dt"="", "formula"=""}], "Output"=[{"Time Values"=[0.0, 0.002, 0.004, 0.006, 0.008, 0.01, 0.012, 0.014, 0.016, 0.018000000000000002, 0.02, 0.022, 0.024, 0.026000000000000002, 0.028, 0.03, 0.032, 0.034, 0.036000000000000004, 0.038, 0.04, 0.042, 0.044, 0.046, 0.048, 0.05, 0.052000000000000005, 0.054, 0.056, 0.058, 0.06, 0.062, 0.064, 0.066, 0.068, 0.07, 0.07200000000000001, 0.074, 0.076, 0.078, 0.08, 0.082, 0.084, 0.08600000000000001, 0.088, 0.09, 0.092, 0.094, 0.096, 0.098, 0.1, 0.10200000000000001, 0.10400000000000001, 0.106, 0.108, 0.11, 0.112, 0.114, 0.116, 0.11800000000000001, 0.12, 0.122, 0.124, 0.126, 0.128, 0.13, 0.132, 0.134, 0.136, 0.138, 0.14, 0.14200000000000002, 0.14400000000000002, 0.146, 0.148, 0.15, 0.152, 0.154, 0.156, 0.158, 0.16, 0.162, 0.164, 0.166, 0.168, 0.17, 0.17200000000000001, 0.17400000000000002, 0.176, 0.178, 0.18, 0.182, 0.184, 0.186, 0.188, 0.19, 0.192, 0.194, 0.196, 0.198, 0.2, 0.6000000000000001, 0.6000000000000001, 0.6002000000000001, 0.6004, 0.6006000000000001, 0.6008000000000001, 0.6010000000000001, 0.6012000000000001, 0.6014, 0.6016000000000001, 0.6018000000000001, 0.6020000000000001, 0.6022000000000001, 0.6024, 0.6026000000000001, 0.6028000000000001, 0.6030000000000001, 0.6032000000000001, 0.6034, 0.6036000000000001, 0.6038000000000001, 0.6040000000000001, 0.6042000000000001, 0.6044, 0.6046000000000001, 0.6048000000000001, 0.6050000000000001, 0.6052000000000001, 0.6054, 0.6056000000000001, 0.6058000000000001, 0.6060000000000001, 0.6062000000000001, 0.6064, 0.6066000000000001, 0.6068000000000001, 0.6070000000000001, 0.6072000000000001, 0.6074, 0.6076000000000001, 0.6078000000000001, 0.6080000000000001, 0.6082000000000001, 0.6084, 0.6086000000000001, 0.6088000000000001, 0.6090000000000001, 0.6092000000000001, 0.6094, 0.6096000000000001, 0.6098000000000001, 0.6100000000000001, 0.6102000000000001, 0.6104, 0.6106000000000001, 0.6108000000000001, 0.6110000000000001, 0.6112000000000001, 0.6114, 0.6116000000000001, 0.6118000000000001, 0.6120000000000001, 0.6122000000000001, 0.6124, 0.6126, 0.6128000000000001, 0.6130000000000001, 0.6132000000000001, 0.6134000000000001, 0.6136000000000001, 0.6138000000000001, 0.6140000000000001, 0.6142000000000001, 0.6144000000000001, 0.6146, 0.6148000000000001, 0.6150000000000001, 0.6152000000000001, 0.6154000000000001, 0.6156, 0.6158000000000001, 0.6160000000000001, 0.6162000000000001, 0.6164000000000001, 0.6166, 0.6168000000000001, 0.6170000000000001, 0.6172000000000001, 0.6174000000000001, 0.6176, 0.6178000000000001, 0.6180000000000001, 0.6182000000000001, 0.6184000000000001, 0.6186, 0.6188000000000001, 0.6190000000000001, 0.6192000000000001, 0.6194000000000001, 0.6196, 0.6198000000000001, 0.6200000000000001, 0.6202000000000001, 0.6212000000000001], array[205 elements]}, {"Time Values"=[0.0, 0.002, 0.004, 0.006, 0.008, 0.01, 0.012, 0.014, 0.016, 0.018000000000000002, 0.02, 0.022, 0.024, 0.026000000000000002, 0.028, 0.03, 0.032, 0.034, 0.036000000000000004, 0.038, 0.04, 0.042, 0.044, 0.046, 0.048, 0.05, 0.052000000000000005, 0.054, 0.056, 0.058, 0.06, 0.062, 0.064, 0.066, 0.068, 0.07, 0.07200000000000001, 0.074, 0.076, 0.078, 0.08, 0.082, 0.084, 0.08600000000000001, 0.088, 0.09, 0.092, 0.094, 0.096, 0.098, 0.1, 0.10200000000000001, 0.10400000000000001, 0.106, 0.108, 0.11, 0.112, 0.114, 0.116, 0.11800000000000001, 0.12, 0.122, 0.124, 0.126, 0.128, 0.13, 0.132, 0.134, 0.136, 0.138, 0.14, 0.14200000000000002, 0.14400000000000002, 0.146, 0.148, 0.15, 0.152, 0.154, 0.156, 0.158, 0.16, 0.162, 0.164, 0.166, 0.168, 0.17, 0.17200000000000001, 0.17400000000000002, 0.176, 0.178, 0.18, 0.182, 0.184, 0.186, 0.188, 0.19, 0.192, 0.194, 0.196, 0.198, 0.2, 0.6000000000000001, 0.6000000000000001, 0.6002000000000001, 0.6004, 0.6006000000000001, 0.6008000000000001, 0.6010000000000001, 0.6012000000000001, 0.6014, 0.6016000000000001, 0.6018000000000001, 0.6020000000000001, 0.6022000000000001, 0.6024, 0.6026000000000001, 0.6028000000000001, 0.6030000000000001, 0.6032000000000001, 0.6034, 0.6036000000000001, 0.6038000000000001, 0.6040000000000001, 0.6042000000000001, 0.6044, 0.6046000000000001, 0.6048000000000001, 0.6050000000000001, 0.6052000000000001, 0.6054, 0.6056000000000001, 0.6058000000000001, 0.6060000000000001, 0.6062000000000001, 0.6064, 0.6066000000000001, 0.6068000000000001, 0.6070000000000001, 0.6072000000000001, 0.6074, 0.6076000000000001, 0.6078000000000001, 0.6080000000000001, 0.6082000000000001, 0.6084, 0.6086000000000001, 0.6088000000000001, 0.6090000000000001, 0.6092000000000001, 0.6094, 0.6096000000000001, 0.6098000000000001, 0.6100000000000001, 0.6102000000000001, 0.6104, 0.6106000000000001, 0.6108000000000001, 0.6110000000000001, 0.6112000000000001, 0.6114, 0.6116000000000001, 0.6118000000000001, 0.6120000000000001, 0.6122000000000001, 0.6124, 0.6126, 0.6128000000000001, 0.6130000000000001, 0.6132000000000001, 0.6134000000000001, 0.6136000000000001, 0.6138000000000001, 0.6140000000000001, 0.6142000000000001, 0.6144000000000001, 0.6146, 0.6148000000000001, 0.6150000000000001, 0.6152000000000001, 0.6154000000000001, 0.6156, 0.6158000000000001, 0.6160000000000001, 0.6162000000000001, 0.6164000000000001, 0.6166, 0.6168000000000001, 0.6170000000000001, 0.6172000000000001, 0.6174000000000001, 0.6176, 0.6178000000000001, 0.6180000000000001, 0.6182000000000001, 0.6184000000000001, 0.6186, 0.6188000000000001, 0.6190000000000001, 0.6192000000000001, 0.6194000000000001, 0.6196, 0.6198000000000001, 0.6200000000000001, 0.6202000000000001, 0.6212000000000001], array[205 elements]}], "SRS Selection"=enum."1550 Vertical"}, {"lattice ramp"=[{"dt"="", "formula"=""}], "Output"=[{"Time Values"=[0.0, 0.002, 0.004, 0.006, 0.008, 0.01, 0.012, 0.014, 0.016, 0.018000000000000002, 0.02, 0.022, 0.024, 0.026000000000000002, 0.028, 0.03, 0.032, 0.034, 0.036000000000000004, 0.038, 0.04, 0.042, 0.044, 0.046, 0.048, 0.05, 0.052000000000000005, 0.054, 0.056, 0.058, 0.06, 0.062, 0.064, 0.066, 0.068, 0.07, 0.07200000000000001, 0.074, 0.076, 0.078, 0.08, 0.082, 0.084, 0.08600000000000001, 0.088, 0.09, 0.092, 0.094, 0.096, 0.098, 0.1, 0.10200000000000001, 0.10400000000000001, 0.106, 0.108, 0.11, 0.112, 0.114, 0.116, 0.11800000000000001, 0.12, 0.122, 0.124, 0.126, 0.128, 0.13, 0.132, 0.134, 0.136, 0.138, 0.14, 0.14200000000000002, 0.14400000000000002, 0.146, 0.148, 0.15, 0.152, 0.154, 0.156, 0.158, 0.16, 0.162, 0.164, 0.166, 0.168, 0.17, 0.17200000000000001, 0.17400000000000002, 0.176, 0.178, 0.18, 0.182, 0.184, 0.186, 0.188, 0.19, 0.192, 0.194, 0.196, 0.198, 0.2, 0.6000000000000001, 0.6000000000000001, 0.6002000000000001, 0.6004, 0.6006000000000001, 0.6008000000000001, 0.6010000000000001, 0.6012000000000001, 0.6014, 0.6016000000000001, 0.6018000000000001, 0.6020000000000001, 0.6022000000000001, 0.6024, 0.6026000000000001, 0.6028000000000001, 0.6030000000000001, 0.6032000000000001, 0.6034, 0.6036000000000001, 0.6038000000000001, 0.6040000000000001, 0.6042000000000001, 0.6044, 0.6046000000000001, 0.6048000000000001, 0.6050000000000001, 0.6052000000000001, 0.6054, 0.6056000000000001, 0.6058000000000001, 0.6060000000000001, 0.6062000000000001, 0.6064, 0.6066000000000001, 0.6068000000000001, 0.6070000000000001, 0.6072000000000001, 0.6074, 0.6076000000000001, 0.6078000000000001, 0.6080000000000001, 0.6082000000000001, 0.6084, 0.6086000000000001, 0.6088000000000001, 0.6090000000000001, 0.6092000000000001, 0.6094, 0.6096000000000001, 0.6098000000000001, 0.6100000000000001, 0.6102000000000001, 0.6104, 0.6106000000000001, 0.6108000000000001, 0.6110000000000001, 0.6112000000000001, 0.6114, 0.6116000000000001, 0.6118000000000001, 0.6120000000000001, 0.6122000000000001, 0.6124, 0.6126, 0.6128000000000001, 0.6130000000000001, 0.6132000000000001, 0.6134000000000001, 0.6136000000000001, 0.6138000000000001, 0.6140000000000001, 0.6142000000000001, 0.6144000000000001, 0.6146, 0.6148000000000001, 0.6150000000000001, 0.6152000000000001, 0.6154000000000001, 0.6156, 0.6158000000000001, 0.6160000000000001, 0.6162000000000001, 0.6164000000000001, 0.6166, 0.6168000000000001, 0.6170000000000001, 0.6172000000000001, 0.6174000000000001, 0.6176, 0.6178000000000001, 0.6180000000000001, 0.6182000000000001, 0.6184000000000001, 0.6186, 0.6188000000000001, 0.6190000000000001, 0.6192000000000001, 0.6194000000000001, 0.6196, 0.6198000000000001, 0.6200000000000001, 0.6202000000000001, 0.6212000000000001], array[205 elements]}, {"Time Values"=[0.0, 0.002, 0.004, 0.006, 0.008, 0.01, 0.012, 0.014, 0.016, 0.018000000000000002, 0.02, 0.022, 0.024, 0.026000000000000002, 0.028, 0.03, 0.032, 0.034, 0.036000000000000004, 0.038, 0.04, 0.042, 0.044, 0.046, 0.048, 0.05, 0.052000000000000005, 0.054, 0.056, 0.058, 0.06, 0.062, 0.064, 0.066, 0.068, 0.07, 0.07200000000000001, 0.074, 0.076, 0.078, 0.08, 0.082, 0.084, 0.08600000000000001, 0.088, 0.09, 0.092, 0.094, 0.096, 0.098, 0.1, 0.10200000000000001, 0.10400000000000001, 0.106, 0.108, 0.11, 0.112, 0.114, 0.116, 0.11800000000000001, 0.12, 0.122, 0.124, 0.126, 0.128, 0.13, 0.132, 0.134, 0.136, 0.138, 0.14, 0.14200000000000002, 0.14400000000000002, 0.146, 0.148, 0.15, 0.152, 0.154, 0.156, 0.158, 0.16, 0.162, 0.164, 0.166, 0.168, 0.17, 0.17200000000000001, 0.17400000000000002, 0.176, 0.178, 0.18, 0.182, 0.184, 0.186, 0.188, 0.19, 0.192, 0.194, 0.196, 0.198, 0.2, 0.6000000000000001, 0.6000000000000001, 0.6002000000000001, 0.6004, 0.6006000000000001, 0.6008000000000001, 0.6010000000000001, 0.6012000000000001, 0.6014, 0.6016000000000001, 0.6018000000000001, 0.6020000000000001, 0.6022000000000001, 0.6024, 0.6026000000000001, 0.6028000000000001, 0.6030000000000001, 0.6032000000000001, 0.6034, 0.6036000000000001, 0.6038000000000001, 0.6040000000000001, 0.6042000000000001, 0.6044, 0.6046000000000001, 0.6048000000000001, 0.6050000000000001, 0.6052000000000001, 0.6054, 0.6056000000000001, 0.6058000000000001, 0.6060000000000001, 0.6062000000000001, 0.6064, 0.6066000000000001, 0.6068000000000001, 0.6070000000000001, 0.6072000000000001, 0.6074, 0.6076000000000001, 0.6078000000000001, 0.6080000000000001, 0.6082000000000001, 0.6084, 0.6086000000000001, 0.6088000000000001, 0.6090000000000001, 0.6092000000000001, 0.6094, 0.6096000000000001, 0.6098000000000001, 0.6100000000000001, 0.6102000000000001, 0.6104, 0.6106000000000001, 0.6108000000000001, 0.6110000000000001, 0.6112000000000001, 0.6114, 0.6116000000000001, 0.6118000000000001, 0.6120000000000001, 0.6122000000000001, 0.6124, 0.6126, 0.6128000000000001, 0.6130000000000001, 0.6132000000000001, 0.6134000000000001, 0.6136000000000001, 0.6138000000000001, 0.6140000000000001, 0.6142000000000001, 0.6144000000000001, 0.6146, 0.6148000000000001, 0.6150000000000001, 0.6152000000000001, 0.6154000000000001, 0.6156, 0.6158000000000001, 0.6160000000000001, 0.6162000000000001, 0.6164000000000001, 0.6166, 0.6168000000000001, 0.6170000000000001, 0.6172000000000001, 0.6174000000000001, 0.6176, 0.6178000000000001, 0.6180000000000001, 0.6182000000000001, 0.6184000000000001, 0.6186, 0.6188000000000001, 0.6190000000000001, 0.6192000000000001, 0.6194000000000001, 0.6196, 0.6198000000000001, 0.6200000000000001, 0.6202000000000001, 0.6212000000000001], array[205 elements]}], "SRS Selection"=enum."1550 Vertical"}], "Master AO Ramp List"=[{"Ramp index"=10, "Ramp time [s]"="", "Step size [s]"=1000.0, "Ramp Array"=[], "Output Bits"=[]}, {"Ramp index"=10, "Ramp time [s]"="", "Step size [s]"=1000.0, "Ramp Array"=[], "Output Bits"=[]}], "Slave AO Ramp List"=[{"Ramp index"=10, "Ramp time [s]"="", "Step size [s]"=1000.0, "Ramp Array"=[], "Output Bits"=[]}, {"Ramp index"=10, "Ramp time [s]"="", "Step size [s]"=1000.0, "Ramp Array"=[], "Output Bits"=[]}], "Master Novatech Ramp List"=[], "Static Variables"=[]}  # Paramaters
  n1 = Unbundle By Name(w1) -> ("Master PB Staging List"=w20:T3, "Master AO Ramp List"=w19:T4, "Master Novatech Ramp List"=w4:T5, "Slave PB Staging List"=w18:T3, "Slave AO Ramp List"=w17:T4, "Novatech Ramps"=w16:T6, "Sequencing Info"=w15:T7, "SRS Ramps"=w14:T8, "Static Variables"=w3:T9)
  n2 = stacked-sequence {
    tunnel: [_ _ _ _ _ w380] -> w6
    tunnel: [_ _ _ w274 _ _] -> w7
    tunnel: w20 -> [w46 _ _ _ _ _]
    tunnel: w19 -> [w42 _ _ _ _ _]
    tunnel: w18 -> [_ w150 _ _ _ _]
    tunnel: w17 -> [_ w147 _ _ _ _]
    tunnel: w16 -> [_ _ w236 _ _ _]
    tunnel: w15 -> [_ _ _ w275 _ _]
    tunnel: w14 -> [_ _ _ _ _ w368]
    tunnel: [w62 _ _ _ _ _] -> w13
    tunnel: "Path" -> [w51 w167 w234 w278 w330 w371]
    tunnel: [w50 _ _ _ _ _] -> w11
    tunnel: [_ _ w231 _ _ _] -> w8
    tunnel: [_ w166 _ _ _ _] -> w10
    tunnel: [_ w155 _ _ _ _] -> w9
    tunnel: [w23 _ _ _ _ _] -> w5
    tunnel: w4 -> [w24 _ _ _ _ _]
    tunnel: w3 -> [_ _ _ _ w327 _]
    tunnel: [_ _ _ _ w326 _] -> w2
    frame #0 {
      n3 = Strip Path(path=w51) -> (name=w26:string)  [unwired: 1 out]
      "Procedure Name" <- w26
      n4 = Concatenate Strings(w26, "_pb4") -> (w75:string)
      n5 = Concatenate Strings(w26, "_rmp4") -> (w73:string)
      n6 = Concatenate Strings(w26, "_freq4") -> (w40:string)
      n7 = Build Path(base path=w51, name or relative path="master") -> (appended path=w25:path)
      n8 = Build Path(base path=w25, name or relative path=w75) -> (appended path=w49:path)
      n9 = Build Path(base path=w25, name or relative path=w73) -> (appended path=w48:path)
      n10 = Build Path(base path=w25, name or relative path=w40) -> (appended path=w29:path)
      n11 = call <vilib>:"Open_Create_Replace File.vi"("file path"=w49) -> ("error out"=w64:errorcluster, "refnum"=w71:refnum<file>)  [unwired: 5 in, 4 out]
      n12 = call <vilib>:"Open_Create_Replace File.vi"("file path"=w48) -> ("error out"=w53:errorcluster, "refnum"=w60:refnum<file>)  [unwired: 5 in, 4 out]
      n13 = call <vilib>:"Open_Create_Replace File.vi"("file path"=w29) -> ("error out"=w31:errorcluster, "refnum"=w38:refnum<file>)  [unwired: 5 in, 4 out]
      n14 = Get File Size(file=w71, error in=w64) -> (refnum out=w70:refnum<file>, size (in bytes)=w68:i64, 0:w63:errorcluster)
      n15 = Get File Size(file=w60, error in=w53) -> (refnum out=w59:refnum<file>, size (in bytes)=w57:i64, 0:w52:errorcluster)
      n16 = Get File Size(file=w38, error in=w31) -> (refnum out=w37:refnum<file>, size (in bytes)=w35:i64, 0:w30:errorcluster)
      n17 = Unbundle By Name(w63) -> ("status"=w65:bool)
      n18 = Unbundle By Name(w52) -> ("status"=w54:bool)
      n19 = Unbundle By Name(w30) -> ("status"=w32:bool)
      n20 = To Long Integer(number=w68) -> (32bit integer=w69:i32)
      n21 = To Long Integer(number=w57) -> (32bit integer=w58:i32)
      n22 = To Long Integer(number=w35) -> (32bit integer=w36:i32)
      n23 = Equal To 0?(x=w69) -> (x = 0?=w66:bool)
      n24 = Equal To 0?(x=w58) -> (x = 0?=w55:bool)
      n25 = Equal To 0?(x=w36) -> (x = 0?=w33:bool)
      n26 = Index Array(array=w42, index=0) -> (element=w43:T10)
      n27 = Index Array(array=w24, index=0) -> (element=w27:T11)
      n28 = Index Array(array=w46, index=0) -> (element=w45:T12)
      n29 = Or(x=w66, y=w65) -> (x .or. y?=w67:bool)
      n30 = Or(x=w55, y=w54) -> (x .or. y?=w56:bool)
      n31 = Or(x=w33, y=w32) -> (x .or. y?=w34:bool)
      n32 = case shown="False" w67 {
        tunnel: [w129 w146] -> w72
        tunnel: w45 -> [w128 w144]
        tunnel: w70 -> [w127 w146]
        tunnel: [w126 w145] -> w62
        tunnel: w69 -> [w125 _]
        frame False {
          # "Read out each element from the data file"
          n33 = while {
            tunnel: [w140] -> w126 mode=indexing
            tunnel: w128 -> [w139]
            shift-right: [w141] -> w129
            shift-left: w127 -> [w142]
            tunnel: w125 -> [w138]
            shift-right: [w137] -> _
            shift-left: 0 -> [w136]
            stop <- w133 stop-if-true
            n34 = Read from Binary File(5:w139, 11:w142) -> (0:w131:errorcluster, 2:w140:T12, 3:w132:refnum<file>)  [unwired: 1 in, 4 out]
            n35 = Get File Position(4:w131, 7:w132) -> (2:w130:i64, 3:w141:refnum<file>)  [unwired: 1 out]
            n36 = To Long Integer(number=w130) -> (32bit integer=w137:i32)
            n37 = Greater Or Equal?(x=w137, y=w138) -> (x >= y?=w134:bool)
            n38 = Equal?(x=w137, y=w136) -> (x = y?=w135:bool)
            n39 = Or(x=w134, y=w135) -> (x .or. y?=w133:bool)
          }
        }
        frame True {
          n40 = Initialize Array(w144, 0) -> (w145:T3)
        }
      }
      n41 = case shown="False" w56 {
        tunnel: [w106 w123] -> w61
        tunnel: w43 -> [w105 w121]
        tunnel: w59 -> [w104 w123]
        tunnel: [w103 w122] -> w50
        tunnel: w58 -> [w102 _]
        frame False {
          # "Read out each element from the data file"
          n42 = while {
            tunnel: [w117] -> w103 mode=indexing
            tunnel: w105 -> [w116]
            shift-right: [w118] -> w106
            shift-left: w104 -> [w119]
            tunnel: w102 -> [w115]
            shift-right: [w114] -> _
            shift-left: 0 -> [w113]
            stop <- w110 stop-if-true
            n43 = Read from Binary File(5:w116, 11:w119) -> (0:w108:errorcluster, 2:w117:T10, 3:w109:refnum<file>)  [unwired: 1 in, 4 out]
            n44 = Get File Position(4:w108, 7:w109) -> (2:w107:i64, 3:w118:refnum<file>)  [unwired: 1 out]
            n45 = To Long Integer(number=w107) -> (32bit integer=w114:i32)
            n46 = Greater Or Equal?(x=w114, y=w115) -> (x >= y?=w111:bool)
            n47 = Equal?(x=w114, y=w113) -> (x = y?=w112:bool)
            n48 = Or(x=w111, y=w112) -> (x .or. y?=w110:bool)
          }
        }
        frame True {
          n49 = Initialize Array(w121, 0) -> (w122:T4)
        }
      }
      n50 = case shown="False" w34 {
        tunnel: [w83 w100] -> w39
        tunnel: w27 -> [w82 w98]
        tunnel: w37 -> [w81 w100]
        tunnel: [w80 w99] -> w23
        tunnel: w36 -> [w79 _]
        frame False {
          # "Read out each element from the data file"
          n51 = while {
            tunnel: [w94] -> w80 mode=indexing
            tunnel: w82 -> [w93]
            shift-right: [w95] -> w83
            shift-left: w81 -> [w96]
            tunnel: w79 -> [w92]
            shift-right: [w91] -> _
            shift-left: 0 -> [w90]
            stop <- w87 stop-if-true
            n52 = Read from Binary File(5:w93, 11:w96) -> (0:w85:errorcluster, 2:w94:T11, 3:w86:refnum<file>)  [unwired: 1 in, 4 out]
            n53 = Get File Position(4:w85, 7:w86) -> (2:w84:i64, 3:w95:refnum<file>)  [unwired: 1 out]
            n54 = To Long Integer(number=w84) -> (32bit integer=w91:i32)
            n55 = Greater Or Equal?(x=w91, y=w92) -> (x >= y?=w88:bool)
            n56 = Equal?(x=w91, y=w90) -> (x = y?=w89:bool)
            n57 = Or(x=w88, y=w89) -> (x .or. y?=w87:bool)
          }
        }
        frame True {
          n58 = Initialize Array(w98, 0) -> (w99:T5)
        }
      }
      n59 = Close File(refnum=w61) -> ()  [unwired: 1 in, 2 out]
      n60 = Close File(refnum=w39) -> ()  [unwired: 1 in, 2 out]
      n61 = Close File(refnum=w72) -> ()  [unwired: 1 in, 2 out]
    }
    frame #1 {
      n62 = Strip Path(path=w167) -> (name=w178:string)  [unwired: 1 out]
      n63 = Concatenate Strings(w178, "_pb4") -> (w182:string)
      n64 = Concatenate Strings(w178, "_rmp4") -> (w180:string)
      n65 = Build Path(base path=w167, name or relative path="slave") -> (appended path=w179:path)
      n66 = Build Path(base path=w179, name or relative path=w182) -> (appended path=w154:path)
      n67 = Build Path(base path=w179, name or relative path=w180) -> (appended path=w153:path)
      n68 = call <vilib>:"Open_Create_Replace File.vi"("file path"=w154) -> ("error out"=w169:errorcluster, "refnum"=w176:refnum<file>)  [unwired: 5 in, 4 out]
      n69 = call <vilib>:"Open_Create_Replace File.vi"("file path"=w153) -> ("error out"=w157:errorcluster, "refnum"=w164:refnum<file>)  [unwired: 5 in, 4 out]
      n70 = Get File Size(file=w176, error in=w169) -> (refnum out=w175:refnum<file>, size (in bytes)=w173:i64, 0:w168:errorcluster)
      n71 = Get File Size(file=w164, error in=w157) -> (refnum out=w163:refnum<file>, size (in bytes)=w161:i64, 0:w156:errorcluster)
      n72 = Unbundle By Name(w168) -> ("status"=w170:bool)
      n73 = Unbundle By Name(w156) -> ("status"=w158:bool)
      n74 = To Long Integer(number=w173) -> (32bit integer=w174:i32)
      n75 = To Long Integer(number=w161) -> (32bit integer=w162:i32)
      n76 = Equal To 0?(x=w174) -> (x = 0?=w171:bool)
      n77 = Equal To 0?(x=w162) -> (x = 0?=w159:bool)
      n78 = Index Array(array=w150, index=0) -> (element=w151:T12)
      n79 = Index Array(array=w147, index=0) -> (element=w148:T10)
      n80 = Or(x=w171, y=w170) -> (x .or. y?=w172:bool)
      n81 = Or(x=w159, y=w158) -> (x .or. y?=w160:bool)
      n82 = case shown="False" w172 {
        tunnel: [w213 w230] -> w177
        tunnel: w151 -> [w212 w228]
        tunnel: w175 -> [w211 w230]
        tunnel: [w210 w229] -> w166
        tunnel: w174 -> [w209 _]
        frame False {
          # "Read out each element from the data file"
          n83 = while {
            tunnel: [w224] -> w210 mode=indexing
            tunnel: w212 -> [w223]
            shift-right: [w225] -> w213
            shift-left: w211 -> [w226]
            tunnel: w209 -> [w222]
            shift-right: [w221] -> _
            shift-left: 0 -> [w220]
            stop <- w217 stop-if-true
            n84 = Read from Binary File(5:w223, 11:w226) -> (0:w215:errorcluster, 2:w224:T12, 3:w216:refnum<file>)  [unwired: 1 in, 4 out]
            n85 = Get File Position(4:w215, 7:w216) -> (2:w214:i64, 3:w225:refnum<file>)  [unwired: 1 out]
            n86 = To Long Integer(number=w214) -> (32bit integer=w221:i32)
            n87 = Greater Or Equal?(x=w221, y=w222) -> (x >= y?=w218:bool)
            n88 = Equal?(x=w221, y=w220) -> (x = y?=w219:bool)
            n89 = Or(x=w218, y=w219) -> (x .or. y?=w217:bool)
          }
        }
        frame True {
          n90 = Initialize Array(w228, 0) -> (w229:T3)
        }
      }
      n91 = case shown="False" w160 {
        tunnel: [w190 w207] -> w165
        tunnel: w148 -> [w189 w205]
        tunnel: w163 -> [w188 w207]
        tunnel: [w187 w206] -> w155
        tunnel: w162 -> [w186 _]
        frame False {
          # "Read out each element from the data file"
          n92 = while {
            tunnel: [w201] -> w187 mode=indexing
            tunnel: w189 -> [w200]
            shift-right: [w202] -> w190
            shift-left: w188 -> [w203]
            tunnel: w186 -> [w199]
            shift-right: [w198] -> _
            shift-left: 0 -> [w197]
            stop <- w194 stop-if-true
            n93 = Read from Binary File(5:w200, 11:w203) -> (0:w192:errorcluster, 2:w201:T10, 3:w193:refnum<file>)  [unwired: 1 in, 4 out]
            n94 = Get File Position(4:w192, 7:w193) -> (2:w191:i64, 3:w202:refnum<file>)  [unwired: 1 out]
            n95 = To Long Integer(number=w191) -> (32bit integer=w198:i32)
            n96 = Greater Or Equal?(x=w198, y=w199) -> (x >= y?=w195:bool)
            n97 = Equal?(x=w198, y=w197) -> (x = y?=w196:bool)
            n98 = Or(x=w195, y=w196) -> (x .or. y?=w194:bool)
          }
        }
        frame True {
          n99 = Initialize Array(w205, 0) -> (w206:T4)
        }
      }
      n100 = Close File(refnum=w177) -> ()  [unwired: 1 in, 2 out]
      n101 = Close File(refnum=w165) -> ()  [unwired: 1 in, 2 out]
    }
    frame #2 {
      n102 = local read "Procedure Name"() -> (w233:string)
      n103 = Concatenate Strings(w233, "_evp4") -> (w248:string)
      n104 = Build Path(base path=w234, name or relative path=w248) -> (appended path=w237:path)
      n105 = call <vilib>:"Open_Create_Replace File.vi"("file path"=w237) -> ("error out"=w239:errorcluster, "refnum"=w246:refnum<file>)  [unwired: 5 in, 4 out]
      n106 = Get File Size(file=w246, error in=w239) -> (refnum out=w245:refnum<file>, size (in bytes)=w243:i64, 0:w238:errorcluster)
      n107 = Unbundle By Name(w238) -> ("status"=w240:bool)
      n108 = To Long Integer(number=w243) -> (32bit integer=w244:i32)
      n109 = Equal To 0?(x=w244) -> (x = 0?=w241:bool)
      n110 = Index Array(array=w236, index=0) -> (element=w235:T13)
      n111 = Or(x=w241, y=w240) -> (x .or. y?=w242:bool)
      n112 = case shown="False" w242 {
        tunnel: [w255 w272] -> w247
        tunnel: w235 -> [w254 w269]
        tunnel: w245 -> [w253 w272]
        tunnel: [w252 w271] -> w231
        tunnel: w244 -> [w251 _]
        frame False {
          # "Read out each element from the data file"
          n113 = while {
            tunnel: [w266] -> w252 mode=indexing
            tunnel: w254 -> [w265]
            shift-right: [w267] -> w255
            shift-left: w253 -> [w268]
            tunnel: w251 -> [w264]
            shift-right: [w263] -> _
            shift-left: 0 -> [w262]
            stop <- w259 stop-if-true
            n114 = Read from Binary File(5:w265, 11:w268) -> (0:w257:errorcluster, 2:w266:T13, 3:w258:refnum<file>)  [unwired: 1 in, 4 out]
            n115 = Get File Position(4:w257, 7:w258) -> (2:w256:i64, 3:w267:refnum<file>)  [unwired: 1 out]
            n116 = To Long Integer(number=w256) -> (32bit integer=w263:i32)
            n117 = Greater Or Equal?(x=w263, y=w264) -> (x >= y?=w260:bool)
            n118 = Equal?(x=w263, y=w262) -> (x = y?=w261:bool)
            n119 = Or(x=w260, y=w261) -> (x .or. y?=w259:bool)
          }
        }
        frame True {
          n120 = Initialize Array(w269, 0) -> (w271:T6)
        }
      }
      n121 = Close File(refnum=w247) -> ()  [unwired: 1 in, 2 out]
    }
    frame #3 {
      # "Convert to new sequence control"
      n122 = local read "Procedure Name"() -> (w291:string)
      n123 = Concatenate Strings(w291, "_seq4") -> (w288:string)
      n124 = Build Path(base path=w278, name or relative path=w288) -> (appended path=w292:path)
      n125 = call <vilib>:"Open_Create_Replace File.vi"("file path"=w292) -> ("error out"=w280:errorcluster, "refnum"=w287:refnum<file>)  [unwired: 5 in, 4 out]
      n126 = Get File Size(file=w287, error in=w280) -> (refnum out=w286:refnum<file>, size (in bytes)=w284:i64, 0:w279:errorcluster)
      n127 = Unbundle By Name(w279) -> ("status"=w281:bool)
      n128 = To Long Integer(number=w284) -> (32bit integer=w285:i32)
      n129 = Equal To 0?(x=w285) -> (x = 0?=w282:bool)
      n130 = Index Array(array=w275, index=0) -> (element=w276:T14)
      n131 = Or(x=w282, y=w281) -> (x .or. y?=w283:bool)
      n132 = case shown="True" w283 {
        tunnel: [w308 w325] -> w290
        tunnel: w276 -> [w307 w323]
        tunnel: w286 -> [w306 w325]
        tunnel: [w305 w322] -> w273
        tunnel: w285 -> [w304 _]
        frame False {
          # "Read out each element from the data file"
          n133 = while {
            tunnel: [w319] -> w305 mode=indexing
            tunnel: w307 -> [w318]
            shift-right: [w320] -> w308
            shift-left: w306 -> [w321]
            tunnel: w304 -> [w317]
            shift-right: [w316] -> _
            shift-left: 0 -> [w315]
            stop <- w312 stop-if-true
            n134 = Read from Binary File(5:w318, 11:w321) -> (0:w310:errorcluster, 2:w319:T14, 3:w311:refnum<file>)  [unwired: 1 in, 4 out]
            n135 = Get File Position(4:w310, 7:w311) -> (2:w309:i64, 3:w320:refnum<file>)  [unwired: 1 out]
            n136 = To Long Integer(number=w309) -> (32bit integer=w316:i32)
            n137 = Greater Or Equal?(x=w316, y=w317) -> (x >= y?=w313:bool)
            n138 = Equal?(x=w316, y=w315) -> (x = y?=w314:bool)
            n139 = Or(x=w313, y=w314) -> (x .or. y?=w312:bool)
          }
        }
        frame True {
          n140 = Initialize Array(w323, 0) -> (w322:T7)
        }
      }
      n141 = for {
        tunnel: [w294] -> w274 mode=indexing
        tunnel: w273 -> [w293] mode=indexing
        w302 = T15 {"Start"=0.0, "End"=2.11, "Sequenced Data"=[], "Inform\nIgor?"=FALSE, "Computed Step Size"=0.0, "Procedure Variable"="", "Default"=2.11, "Steps"=0}  # Sequencing Info
        n142 = Unbundle By Name(w293) -> ("Start"=w301:dbl, "End"=w300:dbl, "Sequenced Data"=w299:dbl[], "Inform\nIgor?"=w298:bool, "Computed Step Size"=w297:dbl, "Procedure Variable"=w296:string, "Default"=w295:dbl)  [unwired: 1 out]
        n143 = Bundle By Name(cluster=w302, "Start"=w301, "End"=w300, "Sequenced Data"=w299, "Inform\nIgor?"=w298, "Computed Step Size"=w297, "Procedure Variable"=w296, "Default"=w295) -> (w294:T15)
      }
      n144 = Close File(refnum=w290) -> ()  [unwired: 1 in, 2 out]
    }
    frame #4 {
      n145 = local read "Procedure Name"() -> (w343:string)
      n146 = Concatenate Strings(w343, "_var4") -> (w340:string)
      n147 = Build Path(base path=w330, name or relative path=w340) -> (appended path=w344:path)
      n148 = call <vilib>:"Open_Create_Replace File.vi"("file path"=w344) -> ("error out"=w332:errorcluster, "refnum"=w339:refnum<file>)  [unwired: 5 in, 4 out]
      n149 = Get File Size(file=w339, error in=w332) -> (refnum out=w338:refnum<file>, size (in bytes)=w336:i64, 0:w331:errorcluster)
      n150 = Unbundle By Name(w331) -> ("status"=w333:bool)
      n151 = To Long Integer(number=w336) -> (32bit integer=w337:i32)
      n152 = Equal To 0?(x=w337) -> (x = 0?=w334:bool)
      n153 = Index Array(array=w327, index=0) -> (element=w328:T16)
      n154 = Or(x=w334, y=w333) -> (x .or. y?=w335:bool)
      n155 = case shown="True" w335 {
        tunnel: [w350 w367] -> w342
        tunnel: w328 -> [w349 w365]
        tunnel: w338 -> [w348 w367]
        tunnel: [w347 w364] -> w326
        tunnel: w337 -> [w346 _]
        frame False {
          # "Read out each element from the data file"
          n156 = while {
            tunnel: [w361] -> w347 mode=indexing
            tunnel: w349 -> [w360]
            shift-right: [w362] -> w350
            shift-left: w348 -> [w363]
            tunnel: w346 -> [w359]
            shift-right: [w358] -> _
            shift-left: 0 -> [w357]
            stop <- w354 stop-if-true
            n157 = Read from Binary File(5:w360, 11:w363) -> (0:w352:errorcluster, 2:w361:T16, 3:w353:refnum<file>)  [unwired: 1 in, 4 out]
            n158 = Get File Position(4:w352, 7:w353) -> (2:w351:i64, 3:w362:refnum<file>)  [unwired: 1 out]
            n159 = To Long Integer(number=w351) -> (32bit integer=w358:i32)
            n160 = Greater Or Equal?(x=w358, y=w359) -> (x >= y?=w355:bool)
            n161 = Equal?(x=w358, y=w357) -> (x = y?=w356:bool)
            n162 = Or(x=w355, y=w356) -> (x .or. y?=w354:bool)
          }
        }
        frame True {
          n163 = Initialize Array(w365, 0) -> (w364:T9)
        }
      }
      n164 = Close File(refnum=w342) -> ()  [unwired: 1 in, 2 out]
    }
    frame #5 {
      n165 = local read "Procedure Name"() -> (w385:string)
      n166 = Concatenate Strings(w385, "_srs4") -> (w383:string)
      n167 = Build Path(base path=w371, name or relative path=w383) -> (appended path=w386:path)
      n168 = call <vilib>:"Open_Create_Replace File.vi"("file path"=w386) -> ("error out"=w372:errorcluster, "refnum"=w379:refnum<file>)  [unwired: 5 in, 4 out]
      n169 = Get File Size(file=w379, error in=w372) -> (refnum out=w382:refnum<file>, size (in bytes)=w378:i64, 0:w373:errorcluster)
      n170 = Unbundle By Name(w373) -> ("status"=w374:bool)
      n171 = To Long Integer(number=w378) -> (32bit integer=w377:i32)
      n172 = Equal To 0?(x=w377) -> (x = 0?=w375:bool)
      n173 = Index Array(array=w368, index=0) -> (element=w369:T17)
      n174 = Or(x=w375, y=w374) -> (x .or. y?=w376:bool)
      n175 = case shown="False" w376 {
        tunnel: w382 -> [w391 w405]
        tunnel: [w390 w405] -> w381
        tunnel: [w389 w402] -> w380
        tunnel: w369 -> [w388 w403]
        tunnel: w377 -> [w387 _]
        frame False {
          # "Read out each element from the data file"
          n176 = while {
            tunnel: [w399] -> w389 mode=indexing
            tunnel: w388 -> [w398]
            shift-right: [w400] -> w390
            shift-left: w391 -> [w401]
            tunnel: w387 -> [w397]
            stop <- w395 stop-if-true
            n177 = Read from Binary File(5:w398, 11:w401) -> (0:w393:errorcluster, 2:w399:T17, 3:w394:refnum<file>)  [unwired: 1 in, 4 out]
            n178 = Get File Position(4:w393, 7:w394) -> (2:w392:i64, 3:w400:refnum<file>)  [unwired: 1 out]
            n179 = To Long Integer(number=w392) -> (32bit integer=w396:i32)
            n180 = Greater Or Equal?(x=w396, y=w397) -> (x >= y?=w395:bool)
          }
        }
        frame True {
          n181 = Initialize Array(w403, 0) -> (w402:T8)
        }
      }
      n182 = Close File(refnum=w381) -> ()  [unwired: 1 in, 2 out]
    }
  }
  n183 = local read "Paramaters"() -> (w22:T1)
  n184 = Bundle By Name(cluster=w22, "Master PB Staging List"=w13, "Master AO Ramp List"=w11, "Master Novatech Ramp List"=w5, "Novatech Ramps"=w8, "Sequencing Info"=w7, "SRS Ramps"=w6, "Slave PB Staging List"=w10, "Slave AO Ramp List"=w9, "Static Variables"=w2) -> (→"Paramaters":T1)
